vi "FlexDDS-NG_USB_Example.vi"() -> ()   [LabVIEW 2016]
uses:
  <vilib>/Utility/xml.llb/Read From XML File(string).vi
  <vilib>/Utility/xml.llb/Write to XML File(string).vi
panel:
  in  "appended instruction string 5":string="dds reset\rdcp spi:CFR1=0x404000\rdcp spi:CFR2=0x80080\rdcp 0 spi:STP0=0x3FFF0000028F5C29\rdcp 1 spi:STP0=0x3FFF0000028F5C29\rdcp 0 spi:DRL=0x147C0118147BC1DB\rdcp 0 spi:DRSS=0xFFFFFFFF00000003\rdcp 0 spi:DRR=0x2D3E\rdcp 0 update:u-d\rdcp 0 update:+d\rdcp 1 spi:DRL=0x147AE148147AE148\rdcp 1 spi:DRSS=0xFFFFFFFF00000000\rdcp 1 spi:DRR=0xFFFF\rdcp 1 update:u-d\rdcp 1 update:+d\rdcp wait:1h:\rdcp wait::DROVER\rdcp 0 spi:DRL=0x147C51F1147C0118\rdcp 0 spi:DRSS=0xFFFFFFFF00000004\rdcp 0 spi:DRR=0x2F2F\rdcp 0 update:u-d\rdcp 0 update:+d\rdcp wait:1h:\rdcp wait::DROVER\rdcp 0 spi:DRL=0x147CB92D147C51F1\rdcp 0 spi:DRSS=0xFFFFFFFF00000017\rdcp 0 spi:DRR=0xD478\rdcp 0 update:u-d\rdcp 0 update:+d\rdcp wait:1h:\rdcp wait::DROVER\rdcp 0 spi:DRL=0x147D3CCC147CB92D\rdcp 0 spi:DRSS=0xFFFFFFFF00000009\rdcp 0 spi:DRR=0x4136\rdcp 0 update:u-d\rdcp 0 update:+d\rdcp wait:1h:\rdcp wait::DROVER\rdcp 0 spi:DRL=0x147DE446147D3CCC\rdcp 0 spi:DRSS=0xFFFFFFFF0000000D\rdcp 0 spi:DRR=0x4A07\rdcp 0 update:u-d\rdcp 0 update:+d\rdcp wait:1h:\rdcp wait::DROVER\rdcp 0 spi:DRL=0x147EB8D6147DE446\rdcp 0 spi:DRSS=0xFFFFFFFF0000002B\rdcp 0 spi:DRR=0xC0EC\rdcp 0 update:u-d\rdcp 0 update:+d\rdcp wait:1h:\rdcp wait::DROVER\rdcp 0 spi:DRL=0x147FC5C3147EB8D6\rdcp 0 spi:DRSS=0xFFFFFFFF00000006\rdcp 0 spi:DRR=0x1547\rdcp 0 update:u-d\rdcp 0 update:+d\rdcp wait:1h:\rdcp wait::DROVER\rdcp 0 spi:DRL=0x148118A1147FC5C3\rdcp 0 spi:DRSS=0xFFFFFFFF0000001C\rdcp 0 spi:DRR=0x4ECD\rdcp 0 update:u-d\rdcp 0 update:+d\rdcp wait:1h:\rdcp wait::DROVER\rdcp 0 spi:DRL=0x1482C174148118A1\rdcp 0 spi:DRSS=0xFFFFFFFF00000049\rdcp 0 spi:DRR=0xA3E0\rdcp 0 update:u-d\rdcp 0 update:+d\rdcp wait:1h:\rdcp wait::DROVER\rdcp 0 spi:DRL=0x1484D2A81482C174\rdcp 0 spi:DRSS=0xFFFFFFFF00000003\rdcp 0 spi:DRR=0x568\rdcp 0 update:u-d\rdcp 0 update:+d\rdcp wait:1h:\rdcp wait::DROVER\rdcp 0 spi:DRL=0x148760AD1484D2A8\rdcp 0 spi:DRSS=0xFFFFFFFF0000008C\rdcp 0 spi:DRR=0xCC25\rdcp 0 update:u-d\rdcp 0 update:+d\rdcp wait:1h:\rdcp wait::DROVER\rdcp 0 spi:DRL=0x148A8111148760AD\rdcp 0 spi:DRSS=0xFFFFFFFF00000049\rdcp 0 spi:DRR=0x56FB\rdcp 0 update:u-d\rdcp 0 update:+d\rdcp wait:1h:\rdcp wait::DROVER\rdcp 0 spi:DRL=0x148E48EB148A8111\rdcp 0 spi:DRSS=0xFFFFFFFF00000004\rdcp 0 spi:DRR=0x3F1\rdcp 0 update:u-d\rdcp 0 update:+d\rdcp wait:1h:\rdcp wait::DROVER\rdcp 0 spi:DRL=0x1492CA77148E48EB\rdcp 0 spi:DRSS=0xFFFFFFFF000000A0\rdcp 0 spi:DRR=0x8447\rdcp 0 update:u-d\rdcp 0 update:+d\rdcp wait:1h:\rdcp wait::DROVER\rdcp 0 spi:DRL=0x149811DB1492CA77\rdcp 0 spi:DRSS=0xFFFFFFFF000000D0\rdcp 0 spi:DRR=0x92C9\rdcp 0 update:u-d\rdcp 0 update:+d\rdcp wait:1h:\rdcp wait::DROVER\rdcp 0 spi:DRL=0x149E2175149811DB\rdcp 0 spi:DRSS=0xFFFFFFFF00000100\rdcp 0 spi:DRR=0x9D59\rdcp 0 update:u-d\rdcp 0 update:+d\rdcp wait:1h:\rdcp wait::DROVER\rdcp 0 spi:DRL=0x14A4EE42149E2175\rdcp 0 spi:DRSS=0xFFFFFFFF000000C7\rdcp 0 spi:DRR=0x6D05\rdcp 0 update:u-d\rdcp 0 update:+d\rdcp wait:1h:\rdcp wait::DROVER\rdcp 0 spi:DRL=0x14AC5D7114A4EE42\rdcp 0 spi:DRSS=0xFFFFFFFF00000019\rdcp 0 spi:DRR=0xC87\rdcp 0 update:u-d\rdcp 0 update:+d\rdcp wait:1h:\rdcp wait::DROVER\rdcp 0 spi:DRL=0x14B4443314AC5D71\rdcp 0 spi:DRSS=0xFFFFFFFF00000021\rdcp 0 spi:DRR=0xF8F\rdcp 0 update:u-d\rdcp 0 update:+d\rdcp wait:1h:\rdcp wait::DROVER\rdcp 0 spi:DRL=0x14BC6A7F14B44433\rdcp 0 spi:DRSS=0xFFFFFFFF0000014D\rdcp 0 spi:DRR=0x9838\rdcp 0 update:u-d\rdcp 0 update:+d\rdcp wait:1h:\rdcp wait::DROVER\rdcp 0 spi:DRL=0x14C490CB14BC6A7F\rdcp 0 spi:DRSS=0xFFFFFFFF0000014D\rdcp 0 spi:DRR=0x9838\rdcp 0 update:u-d\rdcp 0 update:+d\rdcp wait:1h:\rdcp wait::DROVER\rdcp 0 spi:DRL=0x14CC778D14C490CB\rdcp 0 spi:DRSS=0xFFFFFFFF00000021\rdcp 0 spi:DRR=0xF8F\rdcp 0 update:u-d\rdcp 0 update:+d\rdcp wait:1h:\rdcp wait::DROVER\rdcp 0 spi:DRL=0x14D3E6BC14CC778D\rdcp 0 spi:DRSS=0xFFFFFFFF00000019\rdcp 0 spi:DRR=0xC87\rdcp 0 update:u-d\rdcp 0 update:+d\rdcp wait:1h:\rdcp wait::DROVER\rdcp 0 spi:DRL=0x14DAB38914D3E6BC\rdcp 0 spi:DRSS=0xFFFFFFFF000000C7\rdcp 0 spi:DRR=0x6D05\rdcp 0 update:u-d\rdcp 0 update:+d\rdcp wait:1h:\rdcp wait::DROVER\rdcp 0 spi:DRL=0x14E0C32314DAB389\rdcp 0 spi:DRSS=0xFFFFFFFF00000100\rdcp 0 spi:DRR=0x9D59\rdcp 0 update:u-d\rdcp 0 update:+d\rdcp wait:1h:\rdcp wait::DROVER\rdcp 0 spi:DRL=0x14E60A8714E0C323\rdcp 0 spi:DRSS=0xFFFFFFFF000000D0\rdcp 0 spi:DRR=0x92C9\rdcp 0 update:u-d\rdcp 0 update:+d\rdcp wait:1h:\rdcp wait::DROVER\rdcp 0 spi:DRL=0x14EA8C1314E60A87\rdcp 0 spi:DRSS=0xFFFFFFFF000000A0\rdcp 0 spi:DRR=0x8447\rdcp 0 update:u-d\rdcp 0 update:+d\rdcp wait:1h:\rdcp wait::DROVER\rdcp 0 spi:DRL=0x14EE53ED14EA8C13\rdcp 0 spi:DRSS=0xFFFFFFFF00000004\rdcp 0 spi:DRR=0x3F1\rdcp 0 update:u-d\rdcp 0 update:+d\rdcp wait:1h:\rdcp wait::DROVER\rdcp 0 spi:DRL=0x14F1745114EE53ED\rdcp 0 spi:DRSS=0xFFFFFFFF00000049\rdcp 0 spi:DRR=0x56FB\rdcp 0 update:u-d\rdcp 0 update:+d\rdcp wait:1h:\rdcp wait::DROVER\rdcp 0 spi:DRL=0x14F4025514F17451\rdcp 0 spi:DRSS=0xFFFFFFFF0000008C\rdcp 0 spi:DRR=0xCC25\rdcp 0 update:u-d\rdcp 0 update:+d\rdcp wait:1h:\rdcp wait::DROVER\rdcp 0 spi:DRL=0x14F6138A14F40255\rdcp 0 spi:DRSS=0xFFFFFFFF00000003\rdcp 0 spi:DRR=0x568\rdcp 0 update:u-d\rdcp 0 update:+d\rdcp wait:1h:\rdcp wait::DROVER\rdcp 0 spi:DRL=0x14F7BC5D14F6138A\rdcp 0 spi:DRSS=0xFFFFFFFF00000049\rdcp 0 spi:DRR=0xA3E0\rdcp 0 update:u-d\rdcp 0 update:+d\rdcp wait:1h:\rdcp wait::DROVER\rdcp 0 spi:DRL=0x14F90F3B14F7BC5D\rdcp 0 spi:DRSS=0xFFFFFFFF0000001C\rdcp 0 spi:DRR=0x4ECD\rdcp 0 update:u-d\rdcp 0 update:+d\rdcp wait:1h:\rdcp wait::DROVER\rdcp 0 spi:DRL=0x14FA1C2814F90F3B\rdcp 0 spi:DRSS=0xFFFFFFFF00000006\rdcp 0 spi:DRR=0x1547\rdcp 0 update:u-d\rdcp 0 update:+d\rdcp wait:1h:\rdcp wait::DROVER\rdcp 0 spi:DRL=0x14FAF0B814FA1C28\rdcp 0 spi:DRSS=0xFFFFFFFF0000002B\rdcp 0 spi:DRR=0xC0EC\rdcp 0 update:u-d\rdcp 0 update:+d\rdcp wait:1h:\rdcp wait::DROVER\rdcp 0 spi:DRL=0x14FB983214FAF0B8\rdcp 0 spi:DRSS=0xFFFFFFFF0000000D\rdcp 0 spi:DRR=0x4A07\rdcp 0 update:u-d\rdcp 0 update:+d\rdcp wait:1h:\rdcp wait::DROVER\rdcp 0 spi:DRL=0x14FC1BD114FB9832\rdcp 0 spi:DRSS=0xFFFFFFFF00000009\rdcp 0 spi:DRR=0x4136\rdcp 0 update:u-d\rdcp 0 update:+d\rdcp wait:1h:\rdcp wait::DROVER\rdcp 0 spi:DRL=0x14FC830D14FC1BD1\rdcp 0 spi:DRSS=0xFFFFFFFF00000017\rdcp 0 spi:DRR=0xD478\rdcp 0 update:u-d\rdcp 0 update:+d\rdcp wait:1h:\rdcp wait::DROVER\rdcp 0 spi:DRL=0x14FCD3E614FC830D\rdcp 0 spi:DRSS=0xFFFFFFFF00000004\rdcp 0 spi:DRR=0x2F2F\rdcp 0 update:u-d\rdcp 0 update:+d\rdcp wait:1h:\rdcp wait::DROVER\rdcp 0 spi:DRL=0x14FD132314FCD3E6\rdcp 0 spi:DRSS=0xFFFFFFFF00000003\rdcp 0 spi:DRR=0x2D3E\rdcp 0 update:u-d\rdcp 0 update:+d\rdcp wait:1h:\rdcp wait::DROVER\rdcp 0 spi:DRL=0x14FD448E14FD1323\rdcp 0 spi:DRSS=0xFFFFFFFF00000002\rdcp 0 spi:DRR=0x2699\rdcp 0 update:u-d\rdcp 0 update:+d\rdcp wait:1h:\rdcp wait::DROVER\rdcp start\r"
  out "appended instruction string 4":string="dds reset\rdcp spi:CFR1=0x404000\rdcp spi:CFR2=0x80080\rdcp 0 spi:STP0=0x3FFF0000028F5C29\rdcp 1 spi:STP0=0x3FFF0000028F5C29\rdcp 0 spi:DRL=0x147C0118147BC1DB\rdcp 0 spi:DRSS=0xFFFFFFFF00000003\rdcp 0 spi:DRR=0x2D3E\rdcp 0 update:u-d\rdcp 0 update:+d\rdcp 1 spi:DRL=0x147AE148147AE148\rdcp 1 spi:DRSS=0xFFFFFFFF00000000\rdcp 1 spi:DRR=0xFFFF\rdcp 1 update:u-d\rdcp 1 update:+d\rdcp wait:1h:\rdcp wait::DROVER\rdcp 0 spi:DRL=0x147C51F1147C0118\rdcp 0 spi:DRSS=0xFFFFFFFF00000004\rdcp 0 spi:DRR=0x2F2F\rdcp 0 update:u-d\rdcp 0 update:+d\rdcp wait:1h:\rdcp wait::DROVER\rdcp 0 spi:DRL=0x147CB92D147C51F1\rdcp 0 spi:DRSS=0xFFFFFFFF00000017\rdcp 0 spi:DRR=0xD478\rdcp 0 update:u-d\rdcp 0 update:+d\rdcp wait:1h:\rdcp wait::DROVER\rdcp 0 spi:DRL=0x147D3CCC147CB92D\rdcp 0 spi:DRSS=0xFFFFFFFF00000009\rdcp 0 spi:DRR=0x4136\rdcp 0 update:u-d\rdcp 0 update:+d\rdcp wait:1h:\rdcp wait::DROVER\rdcp 0 spi:DRL=0x147DE446147D3CCC\rdcp 0 spi:DRSS=0xFFFFFFFF0000000D\rdcp 0 spi:DRR=0x4A07\rdcp 0 update:u-d\rdcp 0 update:+d\rdcp wait:1h:\rdcp wait::DROVER\rdcp 0 spi:DRL=0x147EB8D6147DE446\rdcp 0 spi:DRSS=0xFFFFFFFF0000002B\rdcp 0 spi:DRR=0xC0EC\rdcp 0 update:u-d\rdcp 0 update:+d\rdcp wait:1h:\rdcp wait::DROVER\rdcp 0 spi:DRL=0x147FC5C3147EB8D6\rdcp 0 spi:DRSS=0xFFFFFFFF00000006\rdcp 0 spi:DRR=0x1547\rdcp 0 update:u-d\rdcp 0 update:+d\rdcp wait:1h:\rdcp wait::DROVER\rdcp 0 spi:DRL=0x148118A1147FC5C3\rdcp 0 spi:DRSS=0xFFFFFFFF0000001C\rdcp 0 spi:DRR=0x4ECD\rdcp 0 update:u-d\rdcp 0 update:+d\rdcp wait:1h:\rdcp wait::DROVER\rdcp 0 spi:DRL=0x1482C174148118A1\rdcp 0 spi:DRSS=0xFFFFFFFF00000049\rdcp 0 spi:DRR=0xA3E0\rdcp 0 update:u-d\rdcp 0 update:+d\rdcp wait:1h:\rdcp wait::DROVER\rdcp 0 spi:DRL=0x1484D2A81482C174\rdcp 0 spi:DRSS=0xFFFFFFFF00000003\rdcp 0 spi:DRR=0x568\rdcp 0 update:u-d\rdcp 0 update:+d\rdcp wait:1h:\rdcp wait::DROVER\rdcp 0 spi:DRL=0x148760AD1484D2A8\rdcp 0 spi:DRSS=0xFFFFFFFF0000008C\rdcp 0 spi:DRR=0xCC25\rdcp 0 update:u-d\rdcp 0 update:+d\rdcp wait:1h:\rdcp wait::DROVER\rdcp 0 spi:DRL=0x148A8111148760AD\rdcp 0 spi:DRSS=0xFFFFFFFF00000049\rdcp 0 spi:DRR=0x56FB\rdcp 0 update:u-d\rdcp 0 update:+d\rdcp wait:1h:\rdcp wait::DROVER\rdcp 0 spi:DRL=0x148E48EB148A8111\rdcp 0 spi:DRSS=0xFFFFFFFF00000004\rdcp 0 spi:DRR=0x3F1\rdcp 0 update:u-d\rdcp 0 update:+d\rdcp wait:1h:\rdcp wait::DROVER\rdcp 0 spi:DRL=0x1492CA77148E48EB\rdcp 0 spi:DRSS=0xFFFFFFFF000000A0\rdcp 0 spi:DRR=0x8447\rdcp 0 update:u-d\rdcp 0 update:+d\rdcp wait:1h:\rdcp wait::DROVER\rdcp 0 spi:DRL=0x149811DB1492CA77\rdcp 0 spi:DRSS=0xFFFFFFFF000000D0\rdcp 0 spi:DRR=0x92C9\rdcp 0 update:u-d\rdcp 0 update:+d\rdcp wait:1h:\rdcp wait::DROVER\rdcp 0 spi:DRL=0x149E2175149811DB\rdcp 0 spi:DRSS=0xFFFFFFFF00000100\rdcp 0 spi:DRR=0x9D59\rdcp 0 update:u-d\rdcp 0 update:+d\rdcp wait:1h:\rdcp wait::DROVER\rdcp 0 spi:DRL=0x14A4EE42149E2175\rdcp 0 spi:DRSS=0xFFFFFFFF000000C7\rdcp 0 spi:DRR=0x6D05\rdcp 0 update:u-d\rdcp 0 update:+d\rdcp wait:1h:\rdcp wait::DROVER\rdcp 0 spi:DRL=0x14AC5D7114A4EE42\rdcp 0 spi:DRSS=0xFFFFFFFF00000019\rdcp 0 spi:DRR=0xC87\rdcp 0 update:u-d\rdcp 0 update:+d\rdcp wait:1h:\rdcp wait::DROVER\rdcp 0 spi:DRL=0x14B4443314AC5D71\rdcp 0 spi:DRSS=0xFFFFFFFF00000021\rdcp 0 spi:DRR=0xF8F\rdcp 0 update:u-d\rdcp 0 update:+d\rdcp wait:1h:\rdcp wait::DROVER\rdcp 0 spi:DRL=0x14BC6A7F14B44433\rdcp 0 spi:DRSS=0xFFFFFFFF0000014D\rdcp 0 spi:DRR=0x9838\rdcp 0 update:u-d\rdcp 0 update:+d\rdcp wait:1h:\rdcp wait::DROVER\rdcp 0 spi:DRL=0x14C490CB14BC6A7F\rdcp 0 spi:DRSS=0xFFFFFFFF0000014D\rdcp 0 spi:DRR=0x9838\rdcp 0 update:u-d\rdcp 0 update:+d\rdcp wait:1h:\rdcp wait::DROVER\rdcp 0 spi:DRL=0x14CC778D14C490CB\rdcp 0 spi:DRSS=0xFFFFFFFF00000021\rdcp 0 spi:DRR=0xF8F\rdcp 0 update:u-d\rdcp 0 update:+d\rdcp wait:1h:\rdcp wait::DROVER\rdcp 0 spi:DRL=0x14D3E6BC14CC778D\rdcp 0 spi:DRSS=0xFFFFFFFF00000019\rdcp 0 spi:DRR=0xC87\rdcp 0 update:u-d\rdcp 0 update:+d\rdcp wait:1h:\rdcp wait::DROVER\rdcp 0 spi:DRL=0x14DAB38914D3E6BC\rdcp 0 spi:DRSS=0xFFFFFFFF000000C7\rdcp 0 spi:DRR=0x6D05\rdcp 0 update:u-d\rdcp 0 update:+d\rdcp wait:1h:\rdcp wait::DROVER\rdcp 0 spi:DRL=0x14E0C32314DAB389\rdcp 0 spi:DRSS=0xFFFFFFFF00000100\rdcp 0 spi:DRR=0x9D59\rdcp 0 update:u-d\rdcp 0 update:+d\rdcp wait:1h:\rdcp wait::DROVER\rdcp 0 spi:DRL=0x14E60A8714E0C323\rdcp 0 spi:DRSS=0xFFFFFFFF000000D0\rdcp 0 spi:DRR=0x92C9\rdcp 0 update:u-d\rdcp 0 update:+d\rdcp wait:1h:\rdcp wait::DROVER\rdcp 0 spi:DRL=0x14EA8C1314E60A87\rdcp 0 spi:DRSS=0xFFFFFFFF000000A0\rdcp 0 spi:DRR=0x8447\rdcp 0 update:u-d\rdcp 0 update:+d\rdcp wait:1h:\rdcp wait::DROVER\rdcp 0 spi:DRL=0x14EE53ED14EA8C13\rdcp 0 spi:DRSS=0xFFFFFFFF00000004\rdcp 0 spi:DRR=0x3F1\rdcp 0 update:u-d\rdcp 0 update:+d\rdcp wait:1h:\rdcp wait::DROVER\rdcp 0 spi:DRL=0x14F1745114EE53ED\rdcp 0 spi:DRSS=0xFFFFFFFF00000049\rdcp 0 spi:DRR=0x56FB\rdcp 0 update:u-d\rdcp 0 update:+d\rdcp wait:1h:\rdcp wait::DROVER\rdcp 0 spi:DRL=0x14F4025514F17451\rdcp 0 spi:DRSS=0xFFFFFFFF0000008C\rdcp 0 spi:DRR=0xCC25\rdcp 0 update:u-d\rdcp 0 update:+d\rdcp wait:1h:\rdcp wait::DROVER\rdcp 0 spi:DRL=0x14F6138A14F40255\rdcp 0 spi:DRSS=0xFFFFFFFF00000003\rdcp 0 spi:DRR=0x568\rdcp 0 update:u-d\rdcp 0 update:+d\rdcp wait:1h:\rdcp wait::DROVER\rdcp 0 spi:DRL=0x14F7BC5D14F6138A\rdcp 0 spi:DRSS=0xFFFFFFFF00000049\rdcp 0 spi:DRR=0xA3E0\rdcp 0 update:u-d\rdcp 0 update:+d\rdcp wait:1h:\rdcp wait::DROVER\rdcp 0 spi:DRL=0x14F90F3B14F7BC5D\rdcp 0 spi:DRSS=0xFFFFFFFF0000001C\rdcp 0 spi:DRR=0x4ECD\rdcp 0 update:u-d\rdcp 0 update:+d\rdcp wait:1h:\rdcp wait::DROVER\rdcp 0 spi:DRL=0x14FA1C2814F90F3B\rdcp 0 spi:DRSS=0xFFFFFFFF00000006\rdcp 0 spi:DRR=0x1547\rdcp 0 update:u-d\rdcp 0 update:+d\rdcp wait:1h:\rdcp wait::DROVER\rdcp 0 spi:DRL=0x14FAF0B814FA1C28\rdcp 0 spi:DRSS=0xFFFFFFFF0000002B\rdcp 0 spi:DRR=0xC0EC\rdcp 0 update:u-d\rdcp 0 update:+d\rdcp wait:1h:\rdcp wait::DROVER\rdcp 0 spi:DRL=0x14FB983214FAF0B8\rdcp 0 spi:DRSS=0xFFFFFFFF0000000D\rdcp 0 spi:DRR=0x4A07\rdcp 0 update:u-d\rdcp 0 update:+d\rdcp wait:1h:\rdcp wait::DROVER\rdcp 0 spi:DRL=0x14FC1BD114FB9832\rdcp 0 spi:DRSS=0xFFFFFFFF00000009\rdcp 0 spi:DRR=0x4136\rdcp 0 update:u-d\rdcp 0 update:+d\rdcp wait:1h:\rdcp wait::DROVER\rdcp 0 spi:DRL=0x14FC830D14FC1BD1\rdcp 0 spi:DRSS=0xFFFFFFFF00000017\rdcp 0 spi:DRR=0xD478\rdcp 0 update:u-d\rdcp 0 update:+d\rdcp wait:1h:\rdcp wait::DROVER\rdcp 0 spi:DRL=0x14FCD3E614FC830D\rdcp 0 spi:DRSS=0xFFFFFFFF00000004\rdcp 0 spi:DRR=0x2F2F\rdcp 0 update:u-d\rdcp 0 update:+d\rdcp wait:1h:\rdcp wait::DROVER\rdcp 0 spi:DRL=0x14FD132314FCD3E6\rdcp 0 spi:DRSS=0xFFFFFFFF00000003\rdcp 0 spi:DRR=0x2D3E\rdcp 0 update:u-d\rdcp 0 update:+d\rdcp wait:1h:\rdcp wait::DROVER\rdcp 0 spi:DRL=0x14FD448E14FD1323\rdcp 0 spi:DRSS=0xFFFFFFFF00000002\rdcp 0 spi:DRR=0x2699\rdcp 0 update:u-d\rdcp 0 update:+d\rdcp wait:1h:\rdcp wait::DROVER\rdcp start\r"
  in  "appended instruction string 3":string="dds reset\rdcp spi:CFR1=0x404000\rdcp spi:CFR2=0x80080\rdcp 0 spi:STP0=0x3FFF0000028F5C29\rdcp 1 spi:STP0=0x3FFF0000028F5C29\rdcp 0 spi:DRL=0x147C0118147BC1DB\rdcp 0 spi:DRSS=0xFFFFFFFF00000003\rdcp 0 spi:DRR=0x2D3E\rdcp 0 update:u-d\rdcp 0 update:+d\rdcp 1 spi:DRL=0x147AE148147AE148\rdcp 1 spi:DRSS=0xFFFFFFFF00000000\rdcp 1 spi:DRR=0xFFFF\rdcp 1 update:u-d\rdcp 1 update:+d\rdcp wait:1h:\rdcp wait::DROVER\rdcp 0 spi:DRL=0x147C51F1147C0118\rdcp 0 spi:DRSS=0xFFFFFFFF00000004\rdcp 0 spi:DRR=0x2F2F\rdcp 0 update:u-d\rdcp 0 update:+d\rdcp wait:1h:\rdcp wait::DROVER\rdcp 0 spi:DRL=0x147CB92D147C51F1\rdcp 0 spi:DRSS=0xFFFFFFFF00000017\rdcp 0 spi:DRR=0xD478\rdcp 0 update:u-d\rdcp 0 update:+d\rdcp wait:1h:\rdcp wait::DROVER\rdcp 0 spi:DRL=0x147D3CCC147CB92D\rdcp 0 spi:DRSS=0xFFFFFFFF00000009\rdcp 0 spi:DRR=0x4136\rdcp 0 update:u-d\rdcp 0 update:+d\rdcp wait:1h:\rdcp wait::DROVER\rdcp 0 spi:DRL=0x147DE446147D3CCC\rdcp 0 spi:DRSS=0xFFFFFFFF0000000D\rdcp 0 spi:DRR=0x4A07\rdcp 0 update:u-d\rdcp 0 update:+d\rdcp wait:1h:\rdcp wait::DROVER\rdcp 0 spi:DRL=0x147EB8D6147DE446\rdcp 0 spi:DRSS=0xFFFFFFFF0000002B\rdcp 0 spi:DRR=0xC0EC\rdcp 0 update:u-d\rdcp 0 update:+d\rdcp wait:1h:\rdcp wait::DROVER\rdcp 0 spi:DRL=0x147FC5C3147EB8D6\rdcp 0 spi:DRSS=0xFFFFFFFF00000006\rdcp 0 spi:DRR=0x1547\rdcp 0 update:u-d\rdcp 0 update:+d\rdcp wait:1h:\rdcp wait::DROVER\rdcp 0 spi:DRL=0x148118A1147FC5C3\rdcp 0 spi:DRSS=0xFFFFFFFF0000001C\rdcp 0 spi:DRR=0x4ECD\rdcp 0 update:u-d\rdcp 0 update:+d\rdcp wait:1h:\rdcp wait::DROVER\rdcp 0 spi:DRL=0x1482C174148118A1\rdcp 0 spi:DRSS=0xFFFFFFFF00000049\rdcp 0 spi:DRR=0xA3E0\rdcp 0 update:u-d\rdcp 0 update:+d\rdcp wait:1h:\rdcp wait::DROVER\rdcp 0 spi:DRL=0x1484D2A81482C174\rdcp 0 spi:DRSS=0xFFFFFFFF00000003\rdcp 0 spi:DRR=0x568\rdcp 0 update:u-d\rdcp 0 update:+d\rdcp wait:1h:\rdcp wait::DROVER\rdcp 0 spi:DRL=0x148760AD1484D2A8\rdcp 0 spi:DRSS=0xFFFFFFFF0000008C\rdcp 0 spi:DRR=0xCC25\rdcp 0 update:u-d\rdcp 0 update:+d\rdcp wait:1h:\rdcp wait::DROVER\rdcp 0 spi:DRL=0x148A8111148760AD\rdcp 0 spi:DRSS=0xFFFFFFFF00000049\rdcp 0 spi:DRR=0x56FB\rdcp 0 update:u-d\rdcp 0 update:+d\rdcp wait:1h:\rdcp wait::DROVER\rdcp 0 spi:DRL=0x148E48EB148A8111\rdcp 0 spi:DRSS=0xFFFFFFFF00000004\rdcp 0 spi:DRR=0x3F1\rdcp 0 update:u-d\rdcp 0 update:+d\rdcp wait:1h:\rdcp wait::DROVER\rdcp 0 spi:DRL=0x1492CA77148E48EB\rdcp 0 spi:DRSS=0xFFFFFFFF000000A0\rdcp 0 spi:DRR=0x8447\rdcp 0 update:u-d\rdcp 0 update:+d\rdcp wait:1h:\rdcp wait::DROVER\rdcp 0 spi:DRL=0x149811DB1492CA77\rdcp 0 spi:DRSS=0xFFFFFFFF000000D0\rdcp 0 spi:DRR=0x92C9\rdcp 0 update:u-d\rdcp 0 update:+d\rdcp wait:1h:\rdcp wait::DROVER\rdcp 0 spi:DRL=0x149E2175149811DB\rdcp 0 spi:DRSS=0xFFFFFFFF00000100\rdcp 0 spi:DRR=0x9D59\rdcp 0 update:u-d\rdcp 0 update:+d\rdcp wait:1h:\rdcp wait::DROVER\rdcp 0 spi:DRL=0x14A4EE42149E2175\rdcp 0 spi:DRSS=0xFFFFFFFF000000C7\rdcp 0 spi:DRR=0x6D05\rdcp 0 update:u-d\rdcp 0 update:+d\rdcp wait:1h:\rdcp wait::DROVER\rdcp 0 spi:DRL=0x14AC5D7114A4EE42\rdcp 0 spi:DRSS=0xFFFFFFFF00000019\rdcp 0 spi:DRR=0xC87\rdcp 0 update:u-d\rdcp 0 update:+d\rdcp wait:1h:\rdcp wait::DROVER\rdcp 0 spi:DRL=0x14B4443314AC5D71\rdcp 0 spi:DRSS=0xFFFFFFFF00000021\rdcp 0 spi:DRR=0xF8F\rdcp 0 update:u-d\rdcp 0 update:+d\rdcp wait:1h:\rdcp wait::DROVER\rdcp 0 spi:DRL=0x14BC6A7F14B44433\rdcp 0 spi:DRSS=0xFFFFFFFF0000014D\rdcp 0 spi:DRR=0x9838\rdcp 0 update:u-d\rdcp 0 update:+d\rdcp wait:1h:\rdcp wait::DROVER\rdcp 0 spi:DRL=0x14C490CB14BC6A7F\rdcp 0 spi:DRSS=0xFFFFFFFF0000014D\rdcp 0 spi:DRR=0x9838\rdcp 0 update:u-d\rdcp 0 update:+d\rdcp wait:1h:\rdcp wait::DROVER\rdcp 0 spi:DRL=0x14CC778D14C490CB\rdcp 0 spi:DRSS=0xFFFFFFFF00000021\rdcp 0 spi:DRR=0xF8F\rdcp 0 update:u-d\rdcp 0 update:+d\rdcp wait:1h:\rdcp wait::DROVER\rdcp 0 spi:DRL=0x14D3E6BC14CC778D\rdcp 0 spi:DRSS=0xFFFFFFFF00000019\rdcp 0 spi:DRR=0xC87\rdcp 0 update:u-d\rdcp 0 update:+d\rdcp wait:1h:\rdcp wait::DROVER\rdcp 0 spi:DRL=0x14DAB38914D3E6BC\rdcp 0 spi:DRSS=0xFFFFFFFF000000C7\rdcp 0 spi:DRR=0x6D05\rdcp 0 update:u-d\rdcp 0 update:+d\rdcp wait:1h:\rdcp wait::DROVER\rdcp 0 spi:DRL=0x14E0C32314DAB389\rdcp 0 spi:DRSS=0xFFFFFFFF00000100\rdcp 0 spi:DRR=0x9D59\rdcp 0 update:u-d\rdcp 0 update:+d\rdcp wait:1h:\rdcp wait::DROVER\rdcp 0 spi:DRL=0x14E60A8714E0C323\rdcp 0 spi:DRSS=0xFFFFFFFF000000D0\rdcp 0 spi:DRR=0x92C9\rdcp 0 update:u-d\rdcp 0 update:+d\rdcp wait:1h:\rdcp wait::DROVER\rdcp 0 spi:DRL=0x14EA8C1314E60A87\rdcp 0 spi:DRSS=0xFFFFFFFF000000A0\rdcp 0 spi:DRR=0x8447\rdcp 0 update:u-d\rdcp 0 update:+d\rdcp wait:1h:\rdcp wait::DROVER\rdcp 0 spi:DRL=0x14EE53ED14EA8C13\rdcp 0 spi:DRSS=0xFFFFFFFF00000004\rdcp 0 spi:DRR=0x3F1\rdcp 0 update:u-d\rdcp 0 update:+d\rdcp wait:1h:\rdcp wait::DROVER\rdcp 0 spi:DRL=0x14F1745114EE53ED\rdcp 0 spi:DRSS=0xFFFFFFFF00000049\rdcp 0 spi:DRR=0x56FB\rdcp 0 update:u-d\rdcp 0 update:+d\rdcp wait:1h:\rdcp wait::DROVER\rdcp 0 spi:DRL=0x14F4025514F17451\rdcp 0 spi:DRSS=0xFFFFFFFF0000008C\rdcp 0 spi:DRR=0xCC25\rdcp 0 update:u-d\rdcp 0 update:+d\rdcp wait:1h:\rdcp wait::DROVER\rdcp 0 spi:DRL=0x14F6138A14F40255\rdcp 0 spi:DRSS=0xFFFFFFFF00000003\rdcp 0 spi:DRR=0x568\rdcp 0 update:u-d\rdcp 0 update:+d\rdcp wait:1h:\rdcp wait::DROVER\rdcp 0 spi:DRL=0x14F7BC5D14F6138A\rdcp 0 spi:DRSS=0xFFFFFFFF00000049\rdcp 0 spi:DRR=0xA3E0\rdcp 0 update:u-d\rdcp 0 update:+d\rdcp wait:1h:\rdcp wait::DROVER\rdcp 0 spi:DRL=0x14F90F3B14F7BC5D\rdcp 0 spi:DRSS=0xFFFFFFFF0000001C\rdcp 0 spi:DRR=0x4ECD\rdcp 0 update:u-d\rdcp 0 update:+d\rdcp wait:1h:\rdcp wait::DROVER\rdcp 0 spi:DRL=0x14FA1C2814F90F3B\rdcp 0 spi:DRSS=0xFFFFFFFF00000006\rdcp 0 spi:DRR=0x1547\rdcp 0 update:u-d\rdcp 0 update:+d\rdcp wait:1h:\rdcp wait::DROVER\rdcp 0 spi:DRL=0x14FAF0B814FA1C28\rdcp 0 spi:DRSS=0xFFFFFFFF0000002B\rdcp 0 spi:DRR=0xC0EC\rdcp 0 update:u-d\rdcp 0 update:+d\rdcp wait:1h:\rdcp wait::DROVER\rdcp 0 spi:DRL=0x14FB983214FAF0B8\rdcp 0 spi:DRSS=0xFFFFFFFF0000000D\rdcp 0 spi:DRR=0x4A07\rdcp 0 update:u-d\rdcp 0 update:+d\rdcp wait:1h:\rdcp wait::DROVER\rdcp 0 spi:DRL=0x14FC1BD114FB9832\rdcp 0 spi:DRSS=0xFFFFFFFF00000009\rdcp 0 spi:DRR=0x4136\rdcp 0 update:u-d\rdcp 0 update:+d\rdcp wait:1h:\rdcp wait::DROVER\rdcp 0 spi:DRL=0x14FC830D14FC1BD1\rdcp 0 spi:DRSS=0xFFFFFFFF00000017\rdcp 0 spi:DRR=0xD478\rdcp 0 update:u-d\rdcp 0 update:+d\rdcp wait:1h:\rdcp wait::DROVER\rdcp 0 spi:DRL=0x14FCD3E614FC830D\rdcp 0 spi:DRSS=0xFFFFFFFF00000004\rdcp 0 spi:DRR=0x2F2F\rdcp 0 update:u-d\rdcp 0 update:+d\rdcp wait:1h:\rdcp wait::DROVER\rdcp 0 spi:DRL=0x14FD132314FCD3E6\rdcp 0 spi:DRSS=0xFFFFFFFF00000003\rdcp 0 spi:DRR=0x2D3E\rdcp 0 update:u-d\rdcp 0 update:+d\rdcp wait:1h:\rdcp wait::DROVER\rdcp 0 spi:DRL=0x14FD448E14FD1323\rdcp 0 spi:DRSS=0xFFFFFFFF00000002\rdcp 0 spi:DRR=0x2699\rdcp 0 update:u-d\rdcp 0 update:+d\rdcp wait:1h:\rdcp wait::DROVER\rdcp start\r"
  in  "Interactive on/off":T1(ring)
  out "return count":u32=6435
  in  "Store data":enum32{"Save settings", "Don't save settings"}(tab)=enum."Don't save settings"
  in  "XML File Path WRITE":path=path "U:/Dokumente/Bachelorarbeit/Labview/FlexDDS-NG/conf/settings_s_curve_up_down.xml"
  in  "Data source":T2(tab)=enum."Generate data with function"
  in  "XML File Path READ":path=path "U:/Dokumente/Bachelorarbeit/Labview/FlexDDS-NG/conf/settings_4consecutive_falling.xml"
  in  "Select curve form":enum32{"S curve", "Exp curve"}(tab)
  in  "s curve parameters":cluster{"k":dbl}={"k"=10.0}
  in  "exp curve parameters":cluster{"k":dbl}={"k"=5.0}
  in  "parameters non-constant channel":T3={"Number of steps"=40, "time [ms]"=10000.0, "start frequency [Hz]"=80000000.0, "end frequency [Hz]"=82000000.0}
  in  "constant frequency":dbl=80000000.0 format="%#_13g"
  in  "Constant Channel":T4(ring)
  in  "CFR2 bits":T5={"Enable ASF from STP (F)"=FALSE, "Digital ramp enable (F)"=TRUE, "Digital ramp no-dwell high (F)"=FALSE, "Digital ramp no-dwell low (F)"=FALSE, "Matched latency enable (T)"=TRUE, "Parallel data port enable (F)"=FALSE}
  in  "CFR1 bits":T6={"RAM enable (F)"=FALSE, "Manual OSK external control (F)"=FALSE, "Inverse sinc filter enable (T)"=TRUE, "DDS sine (/cosine) output (F)"=FALSE, "Load LRR at I/O update (F)"=FALSE, "Autoclear digital ramp accumulator (F)"=TRUE, "Autoclear phase accumulator (F)"=FALSE, "Clear digital ramp accumulator (F)"=FALSE, "Clear phase accumulator (F)"=FALSE, "Load ARR at I/O update (F)"=FALSE, "OSK enable (F)"=FALSE, "Select Auto OSK (F)"=FALSE}
  in  "Trigger before sequence of sweeps":T7(ring)
  in  "appended instruction string 2":string="dds reset\rdcp spi:CFR1=0x404000\rdcp spi:CFR2=0x80080\rdcp 0 spi:STP0=0x3FFF0000028F5C29\rdcp 1 spi:STP0=0x3FFF0000028F5C29\rdcp 0 spi:DRL=0x147C0118147BC1DB\rdcp 0 spi:DRSS=0xFFFFFFFF00000003\rdcp 0 spi:DRR=0x2D3E\rdcp 0 update:u-d\rdcp 0 update:+d\rdcp 1 spi:DRL=0x147AE148147AE148\rdcp 1 spi:DRSS=0xFFFFFFFF00000000\rdcp 1 spi:DRR=0xFFFF\rdcp 1 update:u-d\rdcp 1 update:+d\rdcp wait:1h:\rdcp wait::DROVER\rdcp 0 spi:DRL=0x147C51F1147C0118\rdcp 0 spi:DRSS=0xFFFFFFFF00000004\rdcp 0 spi:DRR=0x2F2F\rdcp 0 update:u-d\rdcp 0 update:+d\rdcp wait:1h:\rdcp wait::DROVER\rdcp 0 spi:DRL=0x147CB92D147C51F1\rdcp 0 spi:DRSS=0xFFFFFFFF00000017\rdcp 0 spi:DRR=0xD478\rdcp 0 update:u-d\rdcp 0 update:+d\rdcp wait:1h:\rdcp wait::DROVER\rdcp 0 spi:DRL=0x147D3CCC147CB92D\rdcp 0 spi:DRSS=0xFFFFFFFF00000009\rdcp 0 spi:DRR=0x4136\rdcp 0 update:u-d\rdcp 0 update:+d\rdcp wait:1h:\rdcp wait::DROVER\rdcp 0 spi:DRL=0x147DE446147D3CCC\rdcp 0 spi:DRSS=0xFFFFFFFF0000000D\rdcp 0 spi:DRR=0x4A07\rdcp 0 update:u-d\rdcp 0 update:+d\rdcp wait:1h:\rdcp wait::DROVER\rdcp 0 spi:DRL=0x147EB8D6147DE446\rdcp 0 spi:DRSS=0xFFFFFFFF0000002B\rdcp 0 spi:DRR=0xC0EC\rdcp 0 update:u-d\rdcp 0 update:+d\rdcp wait:1h:\rdcp wait::DROVER\rdcp 0 spi:DRL=0x147FC5C3147EB8D6\rdcp 0 spi:DRSS=0xFFFFFFFF00000006\rdcp 0 spi:DRR=0x1547\rdcp 0 update:u-d\rdcp 0 update:+d\rdcp wait:1h:\rdcp wait::DROVER\rdcp 0 spi:DRL=0x148118A1147FC5C3\rdcp 0 spi:DRSS=0xFFFFFFFF0000001C\rdcp 0 spi:DRR=0x4ECD\rdcp 0 update:u-d\rdcp 0 update:+d\rdcp wait:1h:\rdcp wait::DROVER\rdcp 0 spi:DRL=0x1482C174148118A1\rdcp 0 spi:DRSS=0xFFFFFFFF00000049\rdcp 0 spi:DRR=0xA3E0\rdcp 0 update:u-d\rdcp 0 update:+d\rdcp wait:1h:\rdcp wait::DROVER\rdcp 0 spi:DRL=0x1484D2A81482C174\rdcp 0 spi:DRSS=0xFFFFFFFF00000003\rdcp 0 spi:DRR=0x568\rdcp 0 update:u-d\rdcp 0 update:+d\rdcp wait:1h:\rdcp wait::DROVER\rdcp 0 spi:DRL=0x148760AD1484D2A8\rdcp 0 spi:DRSS=0xFFFFFFFF0000008C\rdcp 0 spi:DRR=0xCC25\rdcp 0 update:u-d\rdcp 0 update:+d\rdcp wait:1h:\rdcp wait::DROVER\rdcp 0 spi:DRL=0x148A8111148760AD\rdcp 0 spi:DRSS=0xFFFFFFFF00000049\rdcp 0 spi:DRR=0x56FB\rdcp 0 update:u-d\rdcp 0 update:+d\rdcp wait:1h:\rdcp wait::DROVER\rdcp 0 spi:DRL=0x148E48EB148A8111\rdcp 0 spi:DRSS=0xFFFFFFFF00000004\rdcp 0 spi:DRR=0x3F1\rdcp 0 update:u-d\rdcp 0 update:+d\rdcp wait:1h:\rdcp wait::DROVER\rdcp 0 spi:DRL=0x1492CA77148E48EB\rdcp 0 spi:DRSS=0xFFFFFFFF000000A0\rdcp 0 spi:DRR=0x8447\rdcp 0 update:u-d\rdcp 0 update:+d\rdcp wait:1h:\rdcp wait::DROVER\rdcp 0 spi:DRL=0x149811DB1492CA77\rdcp 0 spi:DRSS=0xFFFFFFFF000000D0\rdcp 0 spi:DRR=0x92C9\rdcp 0 update:u-d\rdcp 0 update:+d\rdcp wait:1h:\rdcp wait::DROVER\rdcp 0 spi:DRL=0x149E2175149811DB\rdcp 0 spi:DRSS=0xFFFFFFFF00000100\rdcp 0 spi:DRR=0x9D59\rdcp 0 update:u-d\rdcp 0 update:+d\rdcp wait:1h:\rdcp wait::DROVER\rdcp 0 spi:DRL=0x14A4EE42149E2175\rdcp 0 spi:DRSS=0xFFFFFFFF000000C7\rdcp 0 spi:DRR=0x6D05\rdcp 0 update:u-d\rdcp 0 update:+d\rdcp wait:1h:\rdcp wait::DROVER\rdcp 0 spi:DRL=0x14AC5D7114A4EE42\rdcp 0 spi:DRSS=0xFFFFFFFF00000019\rdcp 0 spi:DRR=0xC87\rdcp 0 update:u-d\rdcp 0 update:+d\rdcp wait:1h:\rdcp wait::DROVER\rdcp 0 spi:DRL=0x14B4443314AC5D71\rdcp 0 spi:DRSS=0xFFFFFFFF00000021\rdcp 0 spi:DRR=0xF8F\rdcp 0 update:u-d\rdcp 0 update:+d\rdcp wait:1h:\rdcp wait::DROVER\rdcp 0 spi:DRL=0x14BC6A7F14B44433\rdcp 0 spi:DRSS=0xFFFFFFFF0000014D\rdcp 0 spi:DRR=0x9838\rdcp 0 update:u-d\rdcp 0 update:+d\rdcp wait:1h:\rdcp wait::DROVER\rdcp 0 spi:DRL=0x14C490CB14BC6A7F\rdcp 0 spi:DRSS=0xFFFFFFFF0000014D\rdcp 0 spi:DRR=0x9838\rdcp 0 update:u-d\rdcp 0 update:+d\rdcp wait:1h:\rdcp wait::DROVER\rdcp 0 spi:DRL=0x14CC778D14C490CB\rdcp 0 spi:DRSS=0xFFFFFFFF00000021\rdcp 0 spi:DRR=0xF8F\rdcp 0 update:u-d\rdcp 0 update:+d\rdcp wait:1h:\rdcp wait::DROVER\rdcp 0 spi:DRL=0x14D3E6BC14CC778D\rdcp 0 spi:DRSS=0xFFFFFFFF00000019\rdcp 0 spi:DRR=0xC87\rdcp 0 update:u-d\rdcp 0 update:+d\rdcp wait:1h:\rdcp wait::DROVER\rdcp 0 spi:DRL=0x14DAB38914D3E6BC\rdcp 0 spi:DRSS=0xFFFFFFFF000000C7\rdcp 0 spi:DRR=0x6D05\rdcp 0 update:u-d\rdcp 0 update:+d\rdcp wait:1h:\rdcp wait::DROVER\rdcp 0 spi:DRL=0x14E0C32314DAB389\rdcp 0 spi:DRSS=0xFFFFFFFF00000100\rdcp 0 spi:DRR=0x9D59\rdcp 0 update:u-d\rdcp 0 update:+d\rdcp wait:1h:\rdcp wait::DROVER\rdcp 0 spi:DRL=0x14E60A8714E0C323\rdcp 0 spi:DRSS=0xFFFFFFFF000000D0\rdcp 0 spi:DRR=0x92C9\rdcp 0 update:u-d\rdcp 0 update:+d\rdcp wait:1h:\rdcp wait::DROVER\rdcp 0 spi:DRL=0x14EA8C1314E60A87\rdcp 0 spi:DRSS=0xFFFFFFFF000000A0\rdcp 0 spi:DRR=0x8447\rdcp 0 update:u-d\rdcp 0 update:+d\rdcp wait:1h:\rdcp wait::DROVER\rdcp 0 spi:DRL=0x14EE53ED14EA8C13\rdcp 0 spi:DRSS=0xFFFFFFFF00000004\rdcp 0 spi:DRR=0x3F1\rdcp 0 update:u-d\rdcp 0 update:+d\rdcp wait:1h:\rdcp wait::DROVER\rdcp 0 spi:DRL=0x14F1745114EE53ED\rdcp 0 spi:DRSS=0xFFFFFFFF00000049\rdcp 0 spi:DRR=0x56FB\rdcp 0 update:u-d\rdcp 0 update:+d\rdcp wait:1h:\rdcp wait::DROVER\rdcp 0 spi:DRL=0x14F4025514F17451\rdcp 0 spi:DRSS=0xFFFFFFFF0000008C\rdcp 0 spi:DRR=0xCC25\rdcp 0 update:u-d\rdcp 0 update:+d\rdcp wait:1h:\rdcp wait::DROVER\rdcp 0 spi:DRL=0x14F6138A14F40255\rdcp 0 spi:DRSS=0xFFFFFFFF00000003\rdcp 0 spi:DRR=0x568\rdcp 0 update:u-d\rdcp 0 update:+d\rdcp wait:1h:\rdcp wait::DROVER\rdcp 0 spi:DRL=0x14F7BC5D14F6138A\rdcp 0 spi:DRSS=0xFFFFFFFF00000049\rdcp 0 spi:DRR=0xA3E0\rdcp 0 update:u-d\rdcp 0 update:+d\rdcp wait:1h:\rdcp wait::DROVER\rdcp 0 spi:DRL=0x14F90F3B14F7BC5D\rdcp 0 spi:DRSS=0xFFFFFFFF0000001C\rdcp 0 spi:DRR=0x4ECD\rdcp 0 update:u-d\rdcp 0 update:+d\rdcp wait:1h:\rdcp wait::DROVER\rdcp 0 spi:DRL=0x14FA1C2814F90F3B\rdcp 0 spi:DRSS=0xFFFFFFFF00000006\rdcp 0 spi:DRR=0x1547\rdcp 0 update:u-d\rdcp 0 update:+d\rdcp wait:1h:\rdcp wait::DROVER\rdcp 0 spi:DRL=0x14FAF0B814FA1C28\rdcp 0 spi:DRSS=0xFFFFFFFF0000002B\rdcp 0 spi:DRR=0xC0EC\rdcp 0 update:u-d\rdcp 0 update:+d\rdcp wait:1h:\rdcp wait::DROVER\rdcp 0 spi:DRL=0x14FB983214FAF0B8\rdcp 0 spi:DRSS=0xFFFFFFFF0000000D\rdcp 0 spi:DRR=0x4A07\rdcp 0 update:u-d\rdcp 0 update:+d\rdcp wait:1h:\rdcp wait::DROVER\rdcp 0 spi:DRL=0x14FC1BD114FB9832\rdcp 0 spi:DRSS=0xFFFFFFFF00000009\rdcp 0 spi:DRR=0x4136\rdcp 0 update:u-d\rdcp 0 update:+d\rdcp wait:1h:\rdcp wait::DROVER\rdcp 0 spi:DRL=0x14FC830D14FC1BD1\rdcp 0 spi:DRSS=0xFFFFFFFF00000017\rdcp 0 spi:DRR=0xD478\rdcp 0 update:u-d\rdcp 0 update:+d\rdcp wait:1h:\rdcp wait::DROVER\rdcp 0 spi:DRL=0x14FCD3E614FC830D\rdcp 0 spi:DRSS=0xFFFFFFFF00000004\rdcp 0 spi:DRR=0x2F2F\rdcp 0 update:u-d\rdcp 0 update:+d\rdcp wait:1h:\rdcp wait::DROVER\rdcp 0 spi:DRL=0x14FD132314FCD3E6\rdcp 0 spi:DRSS=0xFFFFFFFF00000003\rdcp 0 spi:DRR=0x2D3E\rdcp 0 update:u-d\rdcp 0 update:+d\rdcp wait:1h:\rdcp wait::DROVER\rdcp 0 spi:DRL=0x14FD448E14FD1323\rdcp 0 spi:DRSS=0xFFFFFFFF00000002\rdcp 0 spi:DRR=0x2699\rdcp 0 update:u-d\rdcp 0 update:+d\rdcp wait:1h:\rdcp wait::DROVER\rdcp start\r"
  out "frequency-time plot":T8(graph)=[{[{"total time[ms]"=0.0, "f1 [Hz] CH0"=80013385.70184857}, {"total time[ms]"=250.0, "f1 [Hz] CH0"=80017154.97082743}, {"total time[ms]"=250.0, "f1 [Hz] CH0"=80017154.97082743}, {"total time[ms]"=500.0, "f1 [Hz] CH0"=80021973.8852612}, {"total time[ms]"=500.0, "f1 [Hz] CH0"=80021973.8852612}, {"total time[ms]"=750.0, "f1 [Hz] CH0"=80028127.2540865}, {"total time[ms]"=750.0, "f1 [Hz] CH0"=80028127.2540865}, {"total time[ms]"=1000.0, "f1 [Hz] CH0"=80035972.41992418}, {"total time[ms]"=1000.0, "f1 [Hz] CH0"=80035972.41992418}, {"total time[ms]"=1250.0, "f1 [Hz] CH0"=80045954.73982005}, {"total time[ms]"=1250.0, "f1 [Hz] CH0"=80045954.73982005}, {"total time[ms]"=1500.0, "f1 [Hz] CH0"=80058624.46150272}, {"total time[ms]"=1500.0, "f1 [Hz] CH0"=80058624.46150272}, {"total time[ms]"=1750.0, "f1 [Hz] CH0"=80074653.77468826}, {"total time[ms]"=1750.0, "f1 [Hz] CH0"=80074653.77468826}, {"total time[ms]"=2000.0, "f1 [Hz] CH0"=80094851.74635513}, {"total time[ms]"=2000.0, "f1 [Hz] CH0"=80094851.74635513}, {"total time[ms]"=2250.0, "f1 [Hz] CH0"=80120173.30034801}, {"total time[ms]"=2250.0, "f1 [Hz] CH0"=80120173.30034801}, {"total time[ms]"=2500.0, "f1 [Hz] CH0"=80151716.36004248}, {"total time[ms]"=2500.0, "f1 [Hz] CH0"=80151716.36004248}, {"total time[ms]"=2750.0, "f1 [Hz] CH0"=80190698.92979822}, {"total time[ms]"=2750.0, "f1 [Hz] CH0"=80190698.92979822}, {"total time[ms]"=3000.0, "f1 [Hz] CH0"=80238405.84404424}, {"total time[ms]"=3000.0, "f1 [Hz] CH0"=80238405.84404424}, {"total time[ms]"=3250.0, "f1 [Hz] CH0"=80296094.39606337}, {"total time[ms]"=3250.0, "f1 [Hz] CH0"=80296094.39606337}, {"total time[ms]"=3500.0, "f1 [Hz] CH0"=80364851.04761271}, {"total time[ms]"=3500.0, "f1 [Hz] CH0"=80364851.04761271}, {"total time[ms]"=3750.0, "f1 [Hz] CH0"=80445400.27765062}, {"total time[ms]"=3750.0, "f1 [Hz] CH0"=80445400.27765062}, {"total time[ms]"=4000.0, "f1 [Hz] CH0"=80537882.84273998}, {"total time[ms]"=4000.0, "f1 [Hz] CH0"=80537882.84273998}, {"total time[ms]"=4250.0, "f1 [Hz] CH0"=80641642.60164921}, {"total time[ms]"=4250.0, "f1 [Hz] CH0"=80641642.60164921}, {"total time[ms]"=4500.0, "f1 [Hz] CH0"=80755081.3375963}, {"total time[ms]"=4500.0, "f1 [Hz] CH0"=80755081.3375963}, {"total time[ms]"=4750.0, "f1 [Hz] CH0"=80875646.9982284}, {"total time[ms]"=4750.0, "f1 [Hz] CH0"=80875646.9982284}, {"total time[ms]"=5000.0, "f1 [Hz] CH0"=81000000.0}, {"total time[ms]"=5000.0, "f1 [Hz] CH0"=81000000.0}, {"total time[ms]"=5250.0, "f1 [Hz] CH0"=81124353.0017716}, {"total time[ms]"=5250.0, "f1 [Hz] CH0"=81124353.0017716}, {"total time[ms]"=5500.0, "f1 [Hz] CH0"=81244918.6624037}, {"total time[ms]"=5500.0, "f1 [Hz] CH0"=81244918.6624037}, {"total time[ms]"=5750.0, "f1 [Hz] CH0"=81358357.39835079}, {"total time[ms]"=5750.0, "f1 [Hz] CH0"=81358357.39835079}, {"total time[ms]"=6000.0, "f1 [Hz] CH0"=81462117.15726002}, {"total time[ms]"=6000.0, "f1 [Hz] CH0"=81462117.15726002}, {"total time[ms]"=6250.0, "f1 [Hz] CH0"=81554599.72234938}, {"total time[ms]"=6250.0, "f1 [Hz] CH0"=81554599.72234938}, {"total time[ms]"=6500.0, "f1 [Hz] CH0"=81635148.95238729}, {"total time[ms]"=6500.0, "f1 [Hz] CH0"=81635148.95238729}, {"total time[ms]"=6750.0, "f1 [Hz] CH0"=81703905.60393663}, {"total time[ms]"=6750.0, "f1 [Hz] CH0"=81703905.60393663}, {"total time[ms]"=7000.0, "f1 [Hz] CH0"=81761594.15595576}, {"total time[ms]"=7000.0, "f1 [Hz] CH0"=81761594.15595576}, {"total time[ms]"=7250.0, "f1 [Hz] CH0"=81809301.07020178}, {"total time[ms]"=7250.0, "f1 [Hz] CH0"=81809301.07020178}, {"total time[ms]"=7500.0, "f1 [Hz] CH0"=81848283.63995752}, {"total time[ms]"=7500.0, "f1 [Hz] CH0"=81848283.63995752}, {"total time[ms]"=7750.0, "f1 [Hz] CH0"=81879826.69965199}, {"total time[ms]"=7750.0, "f1 [Hz] CH0"=81879826.69965199}, {"total time[ms]"=8000.0, "f1 [Hz] CH0"=81905148.25364487}, {"total time[ms]"=8000.0, "f1 [Hz] CH0"=81905148.25364487}, {"total time[ms]"=8250.0, "f1 [Hz] CH0"=81925346.22531174}, {"total time[ms]"=8250.0, "f1 [Hz] CH0"=81925346.22531174}, {"total time[ms]"=8500.0, "f1 [Hz] CH0"=81941375.53849728}, {"total time[ms]"=8500.0, "f1 [Hz] CH0"=81941375.53849728}, {"total time[ms]"=8750.0, "f1 [Hz] CH0"=81954045.26017995}, {"total time[ms]"=8750.0, "f1 [Hz] CH0"=81954045.26017995}, {"total time[ms]"=9000.0, "f1 [Hz] CH0"=81964027.58007582}, {"total time[ms]"=9000.0, "f1 [Hz] CH0"=81964027.58007582}, {"total time[ms]"=9250.0, "f1 [Hz] CH0"=81971872.7459135}, {"total time[ms]"=9250.0, "f1 [Hz] CH0"=81971872.7459135}, {"total time[ms]"=9500.0, "f1 [Hz] CH0"=81978026.1147388}, {"total time[ms]"=9500.0, "f1 [Hz] CH0"=81978026.1147388}, {"total time[ms]"=9750.0, "f1 [Hz] CH0"=81982845.02917257}, {"total time[ms]"=9750.0, "f1 [Hz] CH0"=81982845.02917257}, {"total time[ms]"=10000.0, "f1 [Hz] CH0"=81986614.29815143}, {"total time[ms]"=10000.0, "f1 [Hz] CH0"=81986614.29815143}, {"total time[ms]"=10250.0, "f1 [Hz] CH0"=81989559.74861288}]}, {[{"total time[ms]"=0.0, "f1 [Hz] CH0"=80000000.0}, {"total time[ms]"=250.0, "f1 [Hz] CH0"=80000000.0}, {"total time[ms]"=250.0, "f1 [Hz] CH0"=80000000.0}, {"total time[ms]"=500.0, "f1 [Hz] CH0"=80000000.0}, {"total time[ms]"=500.0, "f1 [Hz] CH0"=80000000.0}, {"total time[ms]"=750.0, "f1 [Hz] CH0"=80000000.0}, {"total time[ms]"=750.0, "f1 [Hz] CH0"=80000000.0}, {"total time[ms]"=1000.0, "f1 [Hz] CH0"=80000000.0}, {"total time[ms]"=1000.0, "f1 [Hz] CH0"=80000000.0}, {"total time[ms]"=1250.0, "f1 [Hz] CH0"=80000000.0}, {"total time[ms]"=1250.0, "f1 [Hz] CH0"=80000000.0}, {"total time[ms]"=1500.0, "f1 [Hz] CH0"=80000000.0}, {"total time[ms]"=1500.0, "f1 [Hz] CH0"=80000000.0}, {"total time[ms]"=1750.0, "f1 [Hz] CH0"=80000000.0}, {"total time[ms]"=1750.0, "f1 [Hz] CH0"=80000000.0}, {"total time[ms]"=2000.0, "f1 [Hz] CH0"=80000000.0}, {"total time[ms]"=2000.0, "f1 [Hz] CH0"=80000000.0}, {"total time[ms]"=2250.0, "f1 [Hz] CH0"=80000000.0}, {"total time[ms]"=2250.0, "f1 [Hz] CH0"=80000000.0}, {"total time[ms]"=2500.0, "f1 [Hz] CH0"=80000000.0}, {"total time[ms]"=2500.0, "f1 [Hz] CH0"=80000000.0}, {"total time[ms]"=2750.0, "f1 [Hz] CH0"=80000000.0}, {"total time[ms]"=2750.0, "f1 [Hz] CH0"=80000000.0}, {"total time[ms]"=3000.0, "f1 [Hz] CH0"=80000000.0}, {"total time[ms]"=3000.0, "f1 [Hz] CH0"=80000000.0}, {"total time[ms]"=3250.0, "f1 [Hz] CH0"=80000000.0}, {"total time[ms]"=3250.0, "f1 [Hz] CH0"=80000000.0}, {"total time[ms]"=3500.0, "f1 [Hz] CH0"=80000000.0}, {"total time[ms]"=3500.0, "f1 [Hz] CH0"=80000000.0}, {"total time[ms]"=3750.0, "f1 [Hz] CH0"=80000000.0}, {"total time[ms]"=3750.0, "f1 [Hz] CH0"=80000000.0}, {"total time[ms]"=4000.0, "f1 [Hz] CH0"=80000000.0}, {"total time[ms]"=4000.0, "f1 [Hz] CH0"=80000000.0}, {"total time[ms]"=4250.0, "f1 [Hz] CH0"=80000000.0}, {"total time[ms]"=4250.0, "f1 [Hz] CH0"=80000000.0}, {"total time[ms]"=4500.0, "f1 [Hz] CH0"=80000000.0}, {"total time[ms]"=4500.0, "f1 [Hz] CH0"=80000000.0}, {"total time[ms]"=4750.0, "f1 [Hz] CH0"=80000000.0}, {"total time[ms]"=4750.0, "f1 [Hz] CH0"=80000000.0}, {"total time[ms]"=5000.0, "f1 [Hz] CH0"=80000000.0}, {"total time[ms]"=5000.0, "f1 [Hz] CH0"=80000000.0}, {"total time[ms]"=5250.0, "f1 [Hz] CH0"=80000000.0}, {"total time[ms]"=5250.0, "f1 [Hz] CH0"=80000000.0}, {"total time[ms]"=5500.0, "f1 [Hz] CH0"=80000000.0}, {"total time[ms]"=5500.0, "f1 [Hz] CH0"=80000000.0}, {"total time[ms]"=5750.0, "f1 [Hz] CH0"=80000000.0}, {"total time[ms]"=5750.0, "f1 [Hz] CH0"=80000000.0}, {"total time[ms]"=6000.0, "f1 [Hz] CH0"=80000000.0}, {"total time[ms]"=6000.0, "f1 [Hz] CH0"=80000000.0}, {"total time[ms]"=6250.0, "f1 [Hz] CH0"=80000000.0}, {"total time[ms]"=6250.0, "f1 [Hz] CH0"=80000000.0}, {"total time[ms]"=6500.0, "f1 [Hz] CH0"=80000000.0}, {"total time[ms]"=6500.0, "f1 [Hz] CH0"=80000000.0}, {"total time[ms]"=6750.0, "f1 [Hz] CH0"=80000000.0}, {"total time[ms]"=6750.0, "f1 [Hz] CH0"=80000000.0}, {"total time[ms]"=7000.0, "f1 [Hz] CH0"=80000000.0}, {"total time[ms]"=7000.0, "f1 [Hz] CH0"=80000000.0}, {"total time[ms]"=7250.0, "f1 [Hz] CH0"=80000000.0}, {"total time[ms]"=7250.0, "f1 [Hz] CH0"=80000000.0}, {"total time[ms]"=7500.0, "f1 [Hz] CH0"=80000000.0}, {"total time[ms]"=7500.0, "f1 [Hz] CH0"=80000000.0}, {"total time[ms]"=7750.0, "f1 [Hz] CH0"=80000000.0}, {"total time[ms]"=7750.0, "f1 [Hz] CH0"=80000000.0}, {"total time[ms]"=8000.0, "f1 [Hz] CH0"=80000000.0}, {"total time[ms]"=8000.0, "f1 [Hz] CH0"=80000000.0}, {"total time[ms]"=8250.0, "f1 [Hz] CH0"=80000000.0}, {"total time[ms]"=8250.0, "f1 [Hz] CH0"=80000000.0}, {"total time[ms]"=8500.0, "f1 [Hz] CH0"=80000000.0}, {"total time[ms]"=8500.0, "f1 [Hz] CH0"=80000000.0}, {"total time[ms]"=8750.0, "f1 [Hz] CH0"=80000000.0}, {"total time[ms]"=8750.0, "f1 [Hz] CH0"=80000000.0}, {"total time[ms]"=9000.0, "f1 [Hz] CH0"=80000000.0}, {"total time[ms]"=9000.0, "f1 [Hz] CH0"=80000000.0}, {"total time[ms]"=9250.0, "f1 [Hz] CH0"=80000000.0}, {"total time[ms]"=9250.0, "f1 [Hz] CH0"=80000000.0}, {"total time[ms]"=9500.0, "f1 [Hz] CH0"=80000000.0}, {"total time[ms]"=9500.0, "f1 [Hz] CH0"=80000000.0}, {"total time[ms]"=9750.0, "f1 [Hz] CH0"=80000000.0}, {"total time[ms]"=9750.0, "f1 [Hz] CH0"=80000000.0}, {"total time[ms]"=10000.0, "f1 [Hz] CH0"=80000000.0}, {"total time[ms]"=10000.0, "f1 [Hz] CH0"=80000000.0}, {"total time[ms]"=10250.0, "f1 [Hz] CH0"=80000000.0}]}]
  in  "Control Elements Array":T9(array[cluster])=[{"STEP"=0, "time[ms]"=250.0, "time tolerance[us]"=0.01, "CH0"=TRUE, "rel. amplitude CH0"=1.0, "phase [°] CH0"=0.0, "f0 [Hz] CH0"=80013385.70184857, "f1 [Hz] CH0"=80017154.97082743, "CH1"=TRUE, "rel. amplitude CH1"=1.0, "phase [°] CH1"=0.0, "f0 [Hz] CH1"=80000000.0, "f1 [Hz] CH1"=80000000.0}, {"STEP"=0, "time[ms]"=250.0, "time tolerance[us]"=0.01, "CH0"=TRUE, "rel. amplitude CH0"=1.0, "phase [°] CH0"=0.0, "f0 [Hz] CH0"=80017154.97082743, "f1 [Hz] CH0"=80021973.8852612, "CH1"=FALSE, "rel. amplitude CH1"=1.0, "phase [°] CH1"=0.0, "f0 [Hz] CH1"=80000000.0, "f1 [Hz] CH1"=80000000.0}, {"STEP"=0, "time[ms]"=250.0, "time tolerance[us]"=0.01, "CH0"=TRUE, "rel. amplitude CH0"=1.0, "phase [°] CH0"=0.0, "f0 [Hz] CH0"=80021973.8852612, "f1 [Hz] CH0"=80028127.2540865, "CH1"=FALSE, "rel. amplitude CH1"=1.0, "phase [°] CH1"=0.0, "f0 [Hz] CH1"=80000000.0, "f1 [Hz] CH1"=80000000.0}, {"STEP"=0, "time[ms]"=250.0, "time tolerance[us]"=0.01, "CH0"=TRUE, "rel. amplitude CH0"=1.0, "phase [°] CH0"=0.0, "f0 [Hz] CH0"=80028127.2540865, "f1 [Hz] CH0"=80035972.41992418, "CH1"=FALSE, "rel. amplitude CH1"=1.0, "phase [°] CH1"=0.0, "f0 [Hz] CH1"=80000000.0, "f1 [Hz] CH1"=80000000.0}, {"STEP"=0, "time[ms]"=250.0, "time tolerance[us]"=0.01, "CH0"=TRUE, "rel. amplitude CH0"=1.0, "phase [°] CH0"=0.0, "f0 [Hz] CH0"=80035972.41992418, "f1 [Hz] CH0"=80045954.73982005, "CH1"=FALSE, "rel. amplitude CH1"=1.0, "phase [°] CH1"=0.0, "f0 [Hz] CH1"=80000000.0, "f1 [Hz] CH1"=80000000.0}, {"STEP"=0, "time[ms]"=250.0, "time tolerance[us]"=0.01, "CH0"=TRUE, "rel. amplitude CH0"=1.0, "phase [°] CH0"=0.0, "f0 [Hz] CH0"=80045954.73982005, "f1 [Hz] CH0"=80058624.46150272, "CH1"=FALSE, "rel. amplitude CH1"=1.0, "phase [°] CH1"=0.0, "f0 [Hz] CH1"=80000000.0, "f1 [Hz] CH1"=80000000.0}, {"STEP"=0, "time[ms]"=250.0, "time tolerance[us]"=0.01, "CH0"=TRUE, "rel. amplitude CH0"=1.0, "phase [°] CH0"=0.0, "f0 [Hz] CH0"=80058624.46150272, "f1 [Hz] CH0"=80074653.77468826, "CH1"=FALSE, "rel. amplitude CH1"=1.0, "phase [°] CH1"=0.0, "f0 [Hz] CH1"=80000000.0, "f1 [Hz] CH1"=80000000.0}, {"STEP"=0, "time[ms]"=250.0, "time tolerance[us]"=0.01, "CH0"=TRUE, "rel. amplitude CH0"=1.0, "phase [°] CH0"=0.0, "f0 [Hz] CH0"=80074653.77468826, "f1 [Hz] CH0"=80094851.74635513, "CH1"=FALSE, "rel. amplitude CH1"=1.0, "phase [°] CH1"=0.0, "f0 [Hz] CH1"=80000000.0, "f1 [Hz] CH1"=80000000.0}, {"STEP"=0, "time[ms]"=250.0, "time tolerance[us]"=0.01, "CH0"=TRUE, "rel. amplitude CH0"=1.0, "phase [°] CH0"=0.0, "f0 [Hz] CH0"=80094851.74635513, "f1 [Hz] CH0"=80120173.30034801, "CH1"=FALSE, "rel. amplitude CH1"=1.0, "phase [°] CH1"=0.0, "f0 [Hz] CH1"=80000000.0, "f1 [Hz] CH1"=80000000.0}, {"STEP"=0, "time[ms]"=250.0, "time tolerance[us]"=0.01, "CH0"=TRUE, "rel. amplitude CH0"=1.0, "phase [°] CH0"=0.0, "f0 [Hz] CH0"=80120173.30034801, "f1 [Hz] CH0"=80151716.36004248, "CH1"=FALSE, "rel. amplitude CH1"=1.0, "phase [°] CH1"=0.0, "f0 [Hz] CH1"=80000000.0, "f1 [Hz] CH1"=80000000.0}, {"STEP"=0, "time[ms]"=250.0, "time tolerance[us]"=0.01, "CH0"=TRUE, "rel. amplitude CH0"=1.0, "phase [°] CH0"=0.0, "f0 [Hz] CH0"=80151716.36004248, "f1 [Hz] CH0"=80190698.92979822, "CH1"=FALSE, "rel. amplitude CH1"=1.0, "phase [°] CH1"=0.0, "f0 [Hz] CH1"=80000000.0, "f1 [Hz] CH1"=80000000.0}, {"STEP"=0, "time[ms]"=250.0, "time tolerance[us]"=0.01, "CH0"=TRUE, "rel. amplitude CH0"=1.0, "phase [°] CH0"=0.0, "f0 [Hz] CH0"=80190698.92979822, "f1 [Hz] CH0"=80238405.84404424, "CH1"=FALSE, "rel. amplitude CH1"=1.0, "phase [°] CH1"=0.0, "f0 [Hz] CH1"=80000000.0, "f1 [Hz] CH1"=80000000.0}, {"STEP"=0, "time[ms]"=250.0, "time tolerance[us]"=0.01, "CH0"=TRUE, "rel. amplitude CH0"=1.0, "phase [°] CH0"=0.0, "f0 [Hz] CH0"=80238405.84404424, "f1 [Hz] CH0"=80296094.39606337, "CH1"=FALSE, "rel. amplitude CH1"=1.0, "phase [°] CH1"=0.0, "f0 [Hz] CH1"=80000000.0, "f1 [Hz] CH1"=80000000.0}, {"STEP"=0, "time[ms]"=250.0, "time tolerance[us]"=0.01, "CH0"=TRUE, "rel. amplitude CH0"=1.0, "phase [°] CH0"=0.0, "f0 [Hz] CH0"=80296094.39606337, "f1 [Hz] CH0"=80364851.04761271, "CH1"=FALSE, "rel. amplitude CH1"=1.0, "phase [°] CH1"=0.0, "f0 [Hz] CH1"=80000000.0, "f1 [Hz] CH1"=80000000.0}, {"STEP"=0, "time[ms]"=250.0, "time tolerance[us]"=0.01, "CH0"=TRUE, "rel. amplitude CH0"=1.0, "phase [°] CH0"=0.0, "f0 [Hz] CH0"=80364851.04761271, "f1 [Hz] CH0"=80445400.27765062, "CH1"=FALSE, "rel. amplitude CH1"=1.0, "phase [°] CH1"=0.0, "f0 [Hz] CH1"=80000000.0, "f1 [Hz] CH1"=80000000.0}, {"STEP"=0, "time[ms]"=250.0, "time tolerance[us]"=0.01, "CH0"=TRUE, "rel. amplitude CH0"=1.0, "phase [°] CH0"=0.0, "f0 [Hz] CH0"=80445400.27765062, "f1 [Hz] CH0"=80537882.84273998, "CH1"=FALSE, "rel. amplitude CH1"=1.0, "phase [°] CH1"=0.0, "f0 [Hz] CH1"=80000000.0, "f1 [Hz] CH1"=80000000.0}, {"STEP"=0, "time[ms]"=250.0, "time tolerance[us]"=0.01, "CH0"=TRUE, "rel. amplitude CH0"=1.0, "phase [°] CH0"=0.0, "f0 [Hz] CH0"=80537882.84273998, "f1 [Hz] CH0"=80641642.60164921, "CH1"=FALSE, "rel. amplitude CH1"=1.0, "phase [°] CH1"=0.0, "f0 [Hz] CH1"=80000000.0, "f1 [Hz] CH1"=80000000.0}, {"STEP"=0, "time[ms]"=250.0, "time tolerance[us]"=0.01, "CH0"=TRUE, "rel. amplitude CH0"=1.0, "phase [°] CH0"=0.0, "f0 [Hz] CH0"=80641642.60164921, "f1 [Hz] CH0"=80755081.3375963, "CH1"=FALSE, "rel. amplitude CH1"=1.0, "phase [°] CH1"=0.0, "f0 [Hz] CH1"=80000000.0, "f1 [Hz] CH1"=80000000.0}, {"STEP"=0, "time[ms]"=250.0, "time tolerance[us]"=0.01, "CH0"=TRUE, "rel. amplitude CH0"=1.0, "phase [°] CH0"=0.0, "f0 [Hz] CH0"=80755081.3375963, "f1 [Hz] CH0"=80875646.9982284, "CH1"=FALSE, "rel. amplitude CH1"=1.0, "phase [°] CH1"=0.0, "f0 [Hz] CH1"=80000000.0, "f1 [Hz] CH1"=80000000.0}, {"STEP"=0, "time[ms]"=250.0, "time tolerance[us]"=0.01, "CH0"=TRUE, "rel. amplitude CH0"=1.0, "phase [°] CH0"=0.0, "f0 [Hz] CH0"=80875646.9982284, "f1 [Hz] CH0"=81000000.0, "CH1"=FALSE, "rel. amplitude CH1"=1.0, "phase [°] CH1"=0.0, "f0 [Hz] CH1"=80000000.0, "f1 [Hz] CH1"=80000000.0}, {"STEP"=0, "time[ms]"=250.0, "time tolerance[us]"=0.01, "CH0"=TRUE, "rel. amplitude CH0"=1.0, "phase [°] CH0"=0.0, "f0 [Hz] CH0"=81000000.0, "f1 [Hz] CH0"=81124353.0017716, "CH1"=FALSE, "rel. amplitude CH1"=1.0, "phase [°] CH1"=0.0, "f0 [Hz] CH1"=80000000.0, "f1 [Hz] CH1"=80000000.0}, {"STEP"=0, "time[ms]"=250.0, "time tolerance[us]"=0.01, "CH0"=TRUE, "rel. amplitude CH0"=1.0, "phase [°] CH0"=0.0, "f0 [Hz] CH0"=81124353.0017716, "f1 [Hz] CH0"=81244918.6624037, "CH1"=FALSE, "rel. amplitude CH1"=1.0, "phase [°] CH1"=0.0, "f0 [Hz] CH1"=80000000.0, "f1 [Hz] CH1"=80000000.0}, {"STEP"=0, "time[ms]"=250.0, "time tolerance[us]"=0.01, "CH0"=TRUE, "rel. amplitude CH0"=1.0, "phase [°] CH0"=0.0, "f0 [Hz] CH0"=81244918.6624037, "f1 [Hz] CH0"=81358357.39835079, "CH1"=FALSE, "rel. amplitude CH1"=1.0, "phase [°] CH1"=0.0, "f0 [Hz] CH1"=80000000.0, "f1 [Hz] CH1"=80000000.0}, {"STEP"=0, "time[ms]"=250.0, "time tolerance[us]"=0.01, "CH0"=TRUE, "rel. amplitude CH0"=1.0, "phase [°] CH0"=0.0, "f0 [Hz] CH0"=81358357.39835079, "f1 [Hz] CH0"=81462117.15726002, "CH1"=FALSE, "rel. amplitude CH1"=1.0, "phase [°] CH1"=0.0, "f0 [Hz] CH1"=80000000.0, "f1 [Hz] CH1"=80000000.0}, {"STEP"=0, "time[ms]"=250.0, "time tolerance[us]"=0.01, "CH0"=TRUE, "rel. amplitude CH0"=1.0, "phase [°] CH0"=0.0, "f0 [Hz] CH0"=81462117.15726002, "f1 [Hz] CH0"=81554599.72234938, "CH1"=FALSE, "rel. amplitude CH1"=1.0, "phase [°] CH1"=0.0, "f0 [Hz] CH1"=80000000.0, "f1 [Hz] CH1"=80000000.0}, {"STEP"=0, "time[ms]"=250.0, "time tolerance[us]"=0.01, "CH0"=TRUE, "rel. amplitude CH0"=1.0, "phase [°] CH0"=0.0, "f0 [Hz] CH0"=81554599.72234938, "f1 [Hz] CH0"=81635148.95238729, "CH1"=FALSE, "rel. amplitude CH1"=1.0, "phase [°] CH1"=0.0, "f0 [Hz] CH1"=80000000.0, "f1 [Hz] CH1"=80000000.0}, {"STEP"=0, "time[ms]"=250.0, "time tolerance[us]"=0.01, "CH0"=TRUE, "rel. amplitude CH0"=1.0, "phase [°] CH0"=0.0, "f0 [Hz] CH0"=81635148.95238729, "f1 [Hz] CH0"=81703905.60393663, "CH1"=FALSE, "rel. amplitude CH1"=1.0, "phase [°] CH1"=0.0, "f0 [Hz] CH1"=80000000.0, "f1 [Hz] CH1"=80000000.0}, {"STEP"=0, "time[ms]"=250.0, "time tolerance[us]"=0.01, "CH0"=TRUE, "rel. amplitude CH0"=1.0, "phase [°] CH0"=0.0, "f0 [Hz] CH0"=81703905.60393663, "f1 [Hz] CH0"=81761594.15595576, "CH1"=FALSE, "rel. amplitude CH1"=1.0, "phase [°] CH1"=0.0, "f0 [Hz] CH1"=80000000.0, "f1 [Hz] CH1"=80000000.0}, {"STEP"=0, "time[ms]"=250.0, "time tolerance[us]"=0.01, "CH0"=TRUE, "rel. amplitude CH0"=1.0, "phase [°] CH0"=0.0, "f0 [Hz] CH0"=81761594.15595576, "f1 [Hz] CH0"=81809301.07020178, "CH1"=FALSE, "rel. amplitude CH1"=1.0, "phase [°] CH1"=0.0, "f0 [Hz] CH1"=80000000.0, "f1 [Hz] CH1"=80000000.0}, {"STEP"=0, "time[ms]"=250.0, "time tolerance[us]"=0.01, "CH0"=TRUE, "rel. amplitude CH0"=1.0, "phase [°] CH0"=0.0, "f0 [Hz] CH0"=81809301.07020178, "f1 [Hz] CH0"=81848283.63995752, "CH1"=FALSE, "rel. amplitude CH1"=1.0, "phase [°] CH1"=0.0, "f0 [Hz] CH1"=80000000.0, "f1 [Hz] CH1"=80000000.0}, {"STEP"=0, "time[ms]"=250.0, "time tolerance[us]"=0.01, "CH0"=TRUE, "rel. amplitude CH0"=1.0, "phase [°] CH0"=0.0, "f0 [Hz] CH0"=81848283.63995752, "f1 [Hz] CH0"=81879826.69965199, "CH1"=FALSE, "rel. amplitude CH1"=1.0, "phase [°] CH1"=0.0, "f0 [Hz] CH1"=80000000.0, "f1 [Hz] CH1"=80000000.0}, {"STEP"=0, "time[ms]"=250.0, "time tolerance[us]"=0.01, "CH0"=TRUE, "rel. amplitude CH0"=1.0, "phase [°] CH0"=0.0, "f0 [Hz] CH0"=81879826.69965199, "f1 [Hz] CH0"=81905148.25364487, "CH1"=FALSE, "rel. amplitude CH1"=1.0, "phase [°] CH1"=0.0, "f0 [Hz] CH1"=80000000.0, "f1 [Hz] CH1"=80000000.0}, {"STEP"=0, "time[ms]"=250.0, "time tolerance[us]"=0.01, "CH0"=TRUE, "rel. amplitude CH0"=1.0, "phase [°] CH0"=0.0, "f0 [Hz] CH0"=81905148.25364487, "f1 [Hz] CH0"=81925346.22531174, "CH1"=FALSE, "rel. amplitude CH1"=1.0, "phase [°] CH1"=0.0, "f0 [Hz] CH1"=80000000.0, "f1 [Hz] CH1"=80000000.0}, {"STEP"=0, "time[ms]"=250.0, "time tolerance[us]"=0.01, "CH0"=TRUE, "rel. amplitude CH0"=1.0, "phase [°] CH0"=0.0, "f0 [Hz] CH0"=81925346.22531174, "f1 [Hz] CH0"=81941375.53849728, "CH1"=FALSE, "rel. amplitude CH1"=1.0, "phase [°] CH1"=0.0, "f0 [Hz] CH1"=80000000.0, "f1 [Hz] CH1"=80000000.0}, {"STEP"=0, "time[ms]"=250.0, "time tolerance[us]"=0.01, "CH0"=TRUE, "rel. amplitude CH0"=1.0, "phase [°] CH0"=0.0, "f0 [Hz] CH0"=81941375.53849728, "f1 [Hz] CH0"=81954045.26017995, "CH1"=FALSE, "rel. amplitude CH1"=1.0, "phase [°] CH1"=0.0, "f0 [Hz] CH1"=80000000.0, "f1 [Hz] CH1"=80000000.0}, {"STEP"=0, "time[ms]"=250.0, "time tolerance[us]"=0.01, "CH0"=TRUE, "rel. amplitude CH0"=1.0, "phase [°] CH0"=0.0, "f0 [Hz] CH0"=81954045.26017995, "f1 [Hz] CH0"=81964027.58007582, "CH1"=FALSE, "rel. amplitude CH1"=1.0, "phase [°] CH1"=0.0, "f0 [Hz] CH1"=80000000.0, "f1 [Hz] CH1"=80000000.0}, {"STEP"=0, "time[ms]"=250.0, "time tolerance[us]"=0.01, "CH0"=TRUE, "rel. amplitude CH0"=1.0, "phase [°] CH0"=0.0, "f0 [Hz] CH0"=81964027.58007582, "f1 [Hz] CH0"=81971872.7459135, "CH1"=FALSE, "rel. amplitude CH1"=1.0, "phase [°] CH1"=0.0, "f0 [Hz] CH1"=80000000.0, "f1 [Hz] CH1"=80000000.0}, {"STEP"=0, "time[ms]"=250.0, "time tolerance[us]"=0.01, "CH0"=TRUE, "rel. amplitude CH0"=1.0, "phase [°] CH0"=0.0, "f0 [Hz] CH0"=81971872.7459135, "f1 [Hz] CH0"=81978026.1147388, "CH1"=FALSE, "rel. amplitude CH1"=1.0, "phase [°] CH1"=0.0, "f0 [Hz] CH1"=80000000.0, "f1 [Hz] CH1"=80000000.0}, {"STEP"=0, "time[ms]"=250.0, "time tolerance[us]"=0.01, "CH0"=TRUE, "rel. amplitude CH0"=1.0, "phase [°] CH0"=0.0, "f0 [Hz] CH0"=81978026.1147388, "f1 [Hz] CH0"=81982845.02917257, "CH1"=FALSE, "rel. amplitude CH1"=1.0, "phase [°] CH1"=0.0, "f0 [Hz] CH1"=80000000.0, "f1 [Hz] CH1"=80000000.0}, {"STEP"=0, "time[ms]"=250.0, "time tolerance[us]"=0.01, "CH0"=TRUE, "rel. amplitude CH0"=1.0, "phase [°] CH0"=0.0, "f0 [Hz] CH0"=81982845.02917257, "f1 [Hz] CH0"=81986614.29815143, "CH1"=FALSE, "rel. amplitude CH1"=1.0, "phase [°] CH1"=0.0, "f0 [Hz] CH1"=80000000.0, "f1 [Hz] CH1"=80000000.0}, {"STEP"=0, "time[ms]"=250.0, "time tolerance[us]"=0.01, "CH0"=TRUE, "rel. amplitude CH0"=1.0, "phase [°] CH0"=0.0, "f0 [Hz] CH0"=81986614.29815143, "f1 [Hz] CH0"=81989559.74861288, "CH1"=FALSE, "rel. amplitude CH1"=1.0, "phase [°] CH1"=0.0, "f0 [Hz] CH1"=80000000.0, "f1 [Hz] CH1"=80000000.0}]
  out "error out":errorcluster={"status"=TRUE, "code"=-1073807339, "source"="VISA Read in FlexDDS-NG_USB_Example.vi"}
  out "read buffer":string
  in  "FlexDDS-NG USB VISA resource name (COM)":refnum<visa-resource-name>="COM5"
  # "STEP"
  # "time [ms]"
  # "time tolerance [us]"
  # "CH0 [false=wait, keep phase&amplitude]"
  # "rel. amplitude CH0"
  # "phase [°] CH0"
  # "f0 [Hz] CH0"
  # "f1 [Hz] CH0"
  # "CH1 [false=wait, keep phase&amplitude]"
  # "rel. amplitude CH1"
  # "phase [°] CH1"
  # "f0 [Hz] CH1"
  # "f1 [Hz] CH1"
  # "f(t) = f0 + (f1-f0)/(1+exp(-k/Dt * (t-Dt/2)))"
  # "f(t) = f1 - (f1-f0)*exp(-K*t/Dt)"
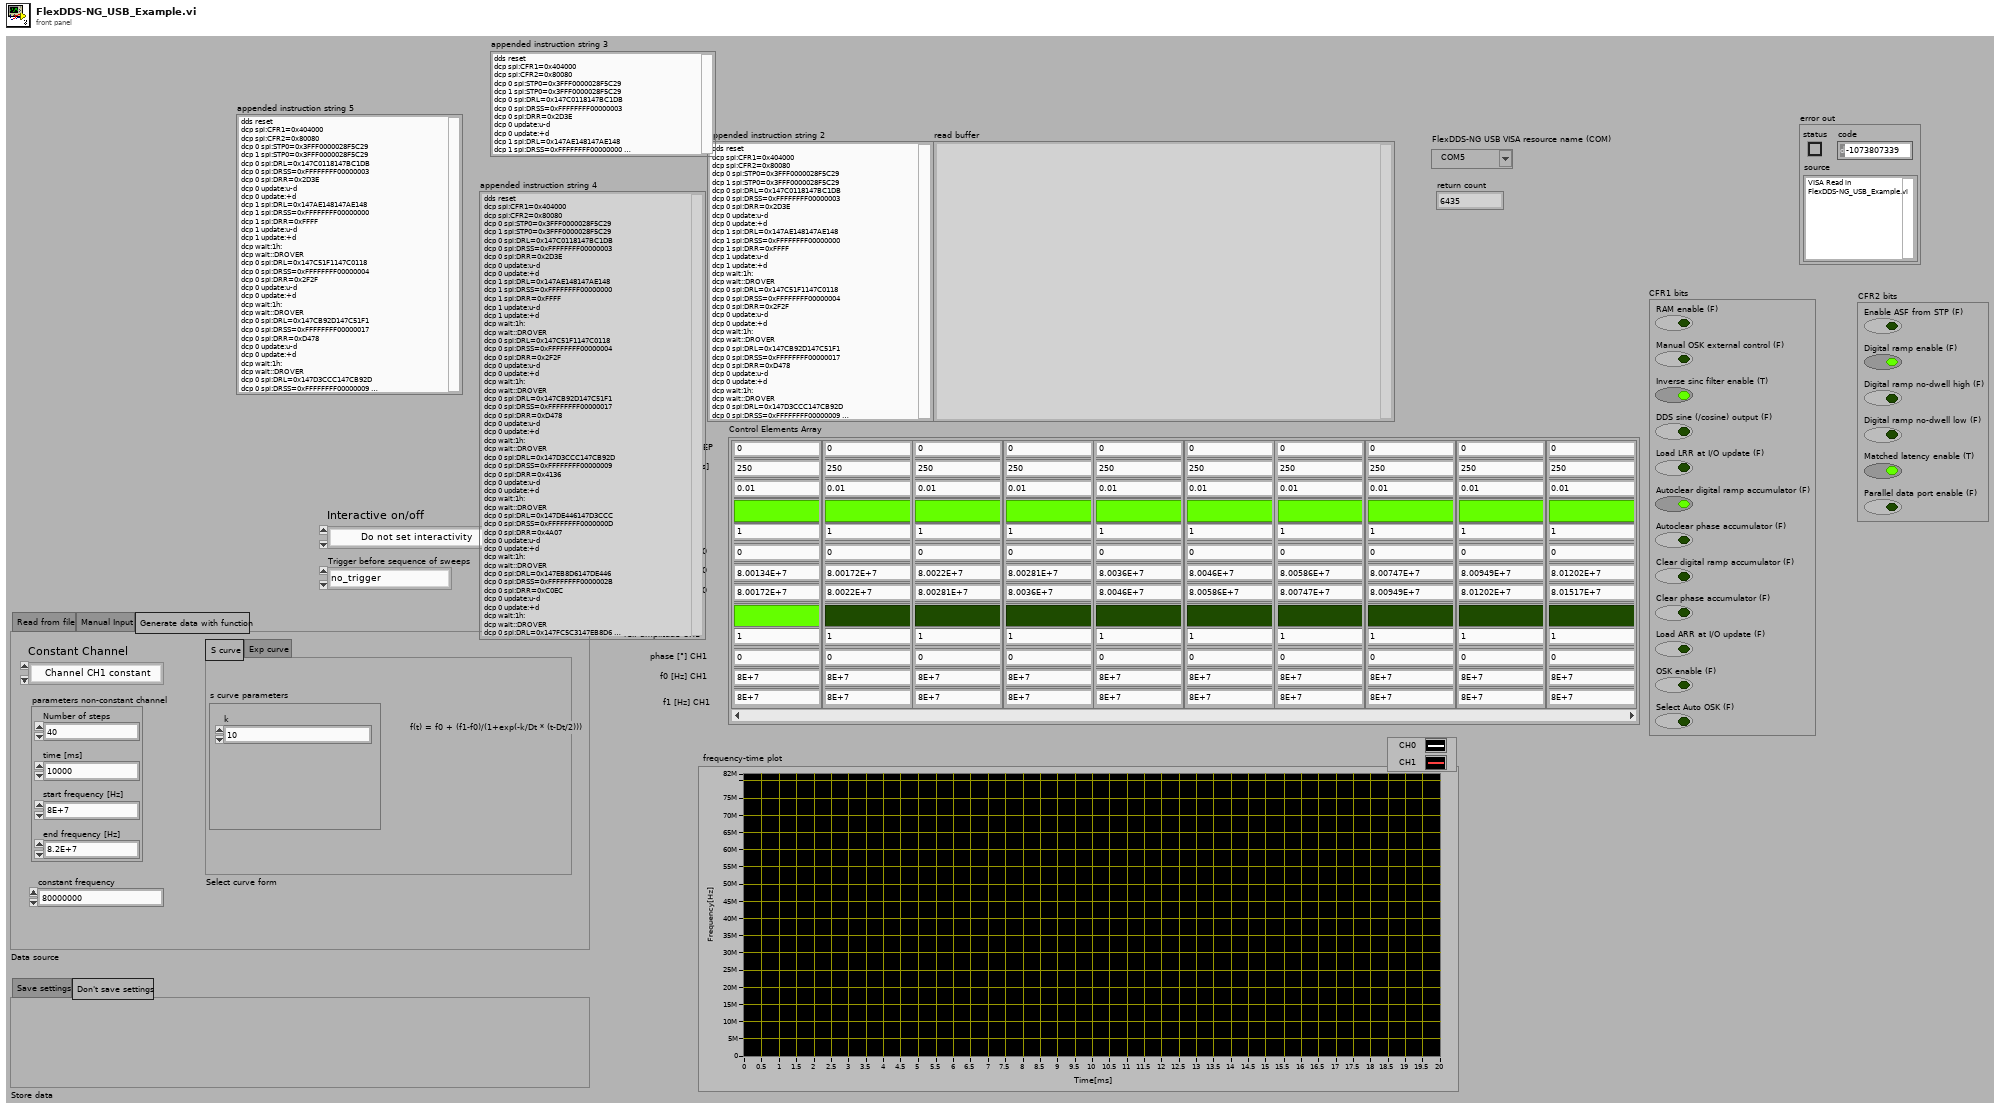
[diagram p1: front panel]
types:
  T1 = enum16{"Do not set interactivity", "Interactive off", "Interactive on"}
  T2 = enum32{"Read from file", "Manual Input", "Generate data with function"}
  T3 = cluster{"Number of steps":i32, "time [ms]":dbl, "start frequency [Hz]":dbl, "end frequency [Hz]":dbl}
  T4 = enum16{"Channel CH1 constant", "Channel CH0 constant"}
  T5 = cluster{"Enable ASF from STP (F)":bool, "Digital ramp enable (F)":bool, "Digital ramp no-dwell high (F)":bool, "Digital ramp no-dwell low (F)":bool, "Matched latency enable (T)":bool, "Parallel data port enable (F)":bool}
  T6 = cluster{"RAM enable (F)":bool, "Manual OSK external control (F)":bool, "Inverse sinc filter enable (T)":bool, "DDS sine (/cosine) output (F)":bool, "Load LRR at I/O update (F)":bool, "Autoclear digital ramp accumulator (F)":bool, "Autoclear phase accumulator (F)":bool, "Clear digital ramp accumulator (F)":bool, "Clear phase accumulator (F)":bool, "Load ARR at I/O update (F)":bool, "OSK enable (F)":bool, "Select Auto OSK (F)":bool}
  T7 = enum16{"no_trigger", "BNC_IN_A_RISING", "BNC_IN_A_FALLING", "BNC_IN_B_RISING", "BNC_IN_B_FALLING", "BNC_IN_C_RISING", "BNC_IN_C_FALLING"}
  T8 = cluster{cluster{"total time[ms]":dbl, "f1 [Hz] CH0":dbl}[]}[]
  T9 = cluster{"STEP":i32, "time[ms]":dbl, "time tolerance[us]":dbl, "CH0":bool, "rel. amplitude CH0":dbl, "phase [°] CH0":dbl, "f0 [Hz] CH0":dbl, "f1 [Hz] CH0":dbl, "CH1":bool, "rel. amplitude CH1":dbl, "phase [°] CH1":dbl, "f0 [Hz] CH1":dbl, "f1 [Hz] CH1":dbl}[]
  T10 = cluster{i32, dbl, "time tolerance":dbl, bool, dbl, dbl, "constant frequency":dbl, "constant frequency":dbl, bool, dbl, dbl, "constant frequency":dbl, "constant frequency":dbl}[]
  T11 = cluster{i32, dbl, "time tolerance":dbl, bool, dbl, dbl, "constant frequency":dbl, "constant frequency":dbl, bool, dbl, dbl, "constant frequency":dbl, "constant frequency":dbl}
  T12 = cluster{"total time[ms]":dbl, "f1 [Hz] CH1":dbl}[]
  T13 = cluster{"total time[ms]":dbl, "f1 [Hz] CH0":dbl}[]
  T14 = cluster{"STEP":i32, "time[ms]":dbl, "time tolerance[us]":dbl, "CH0":bool, "rel. amplitude CH0":dbl, "phase [°] CH0":dbl, "f0 [Hz] CH0":dbl, "f1 [Hz] CH0":dbl, "CH1":bool, "rel. amplitude CH1":dbl, "phase [°] CH1":dbl, "f0 [Hz] CH1":dbl, "f1 [Hz] CH1":dbl}
  T15 = cluster{"Array":cluster{"total time[ms]":dbl, "f1 [Hz] CH0":dbl}[]}
  T16 = cluster{"Array":cluster{"total time[ms]":dbl, "f1 [Hz] CH1":dbl}[]}
  T17 = cluster{"Array":cluster{"total time[ms]":dbl, "f1 [Hz] CH1":dbl}[]}[]
  T18 = enum32{"Channel 0", "Channel 1", "Both channels"}
  T19 = enum32{"O_RAMP_SWP_OVR", "RAM_SWP_OVR", "O_DROVER", "DROVER", "O_SPI_FIFO_EV1", "SPI_FIFO_EV1", "O_SPI_FIFO_EV0", "SPI_FIFO_EV0", "O_SPI_FIFO_FLUSHED", "SPI_FIFO_FLUSHED", "BNC_IN_B_LEVEL", "BNC_IN_B_FALLING", "BNC_IN_B_RISING", "BNC_IN_A_LEVEL", "BNC_IN_A_FALLING", "BNC_IN_A_RISING", "ALL_SPI_FIFOS_FLUSHED", "NONE"}
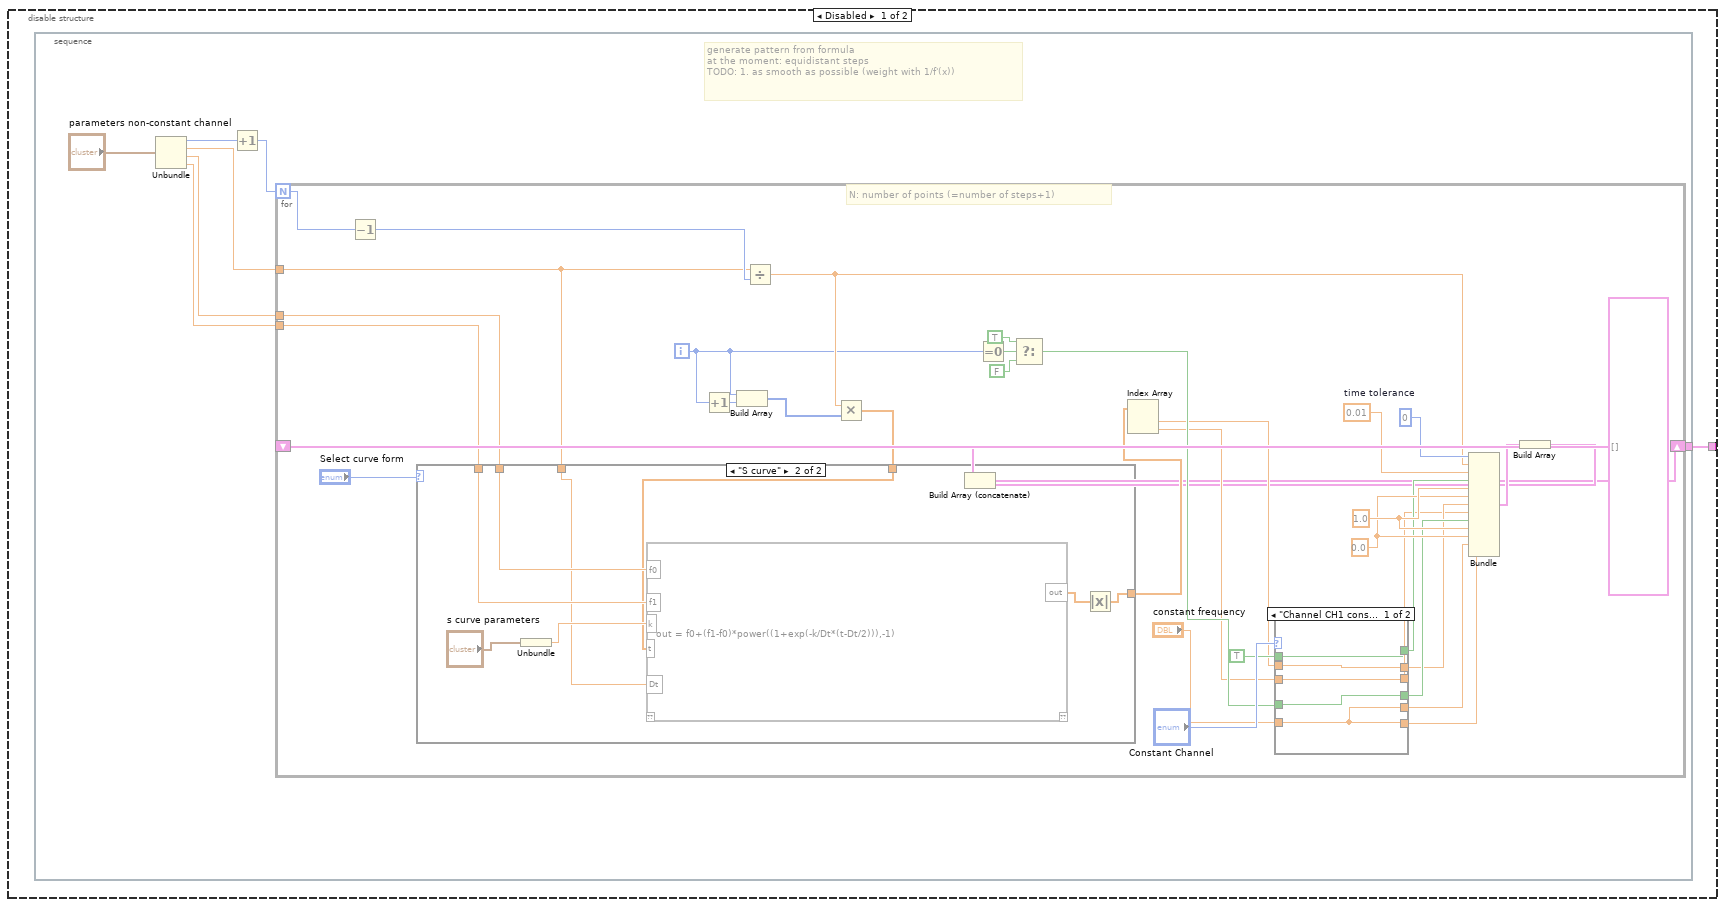
[diagram p2: hidden frame]
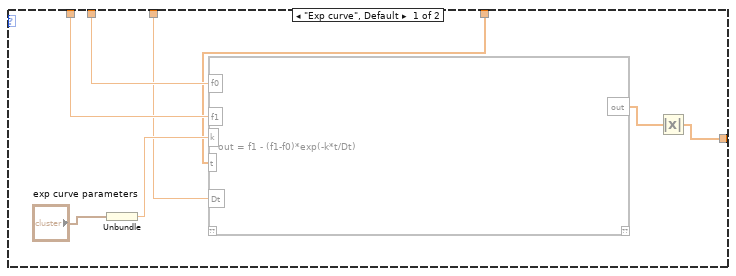
[diagram p4: hidden frame]
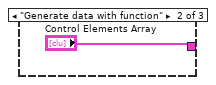
[diagram p5: hidden frame]
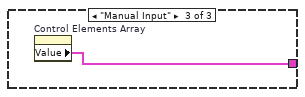
[diagram p6: hidden frame]
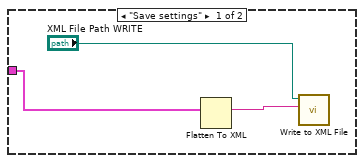
[diagram p7: hidden frame]
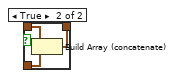
[diagram p8: hidden frame]
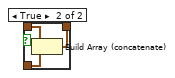
[diagram p9: hidden frame]
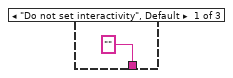
[diagram p10: hidden frame]
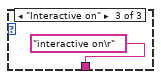
[diagram p11: hidden frame]
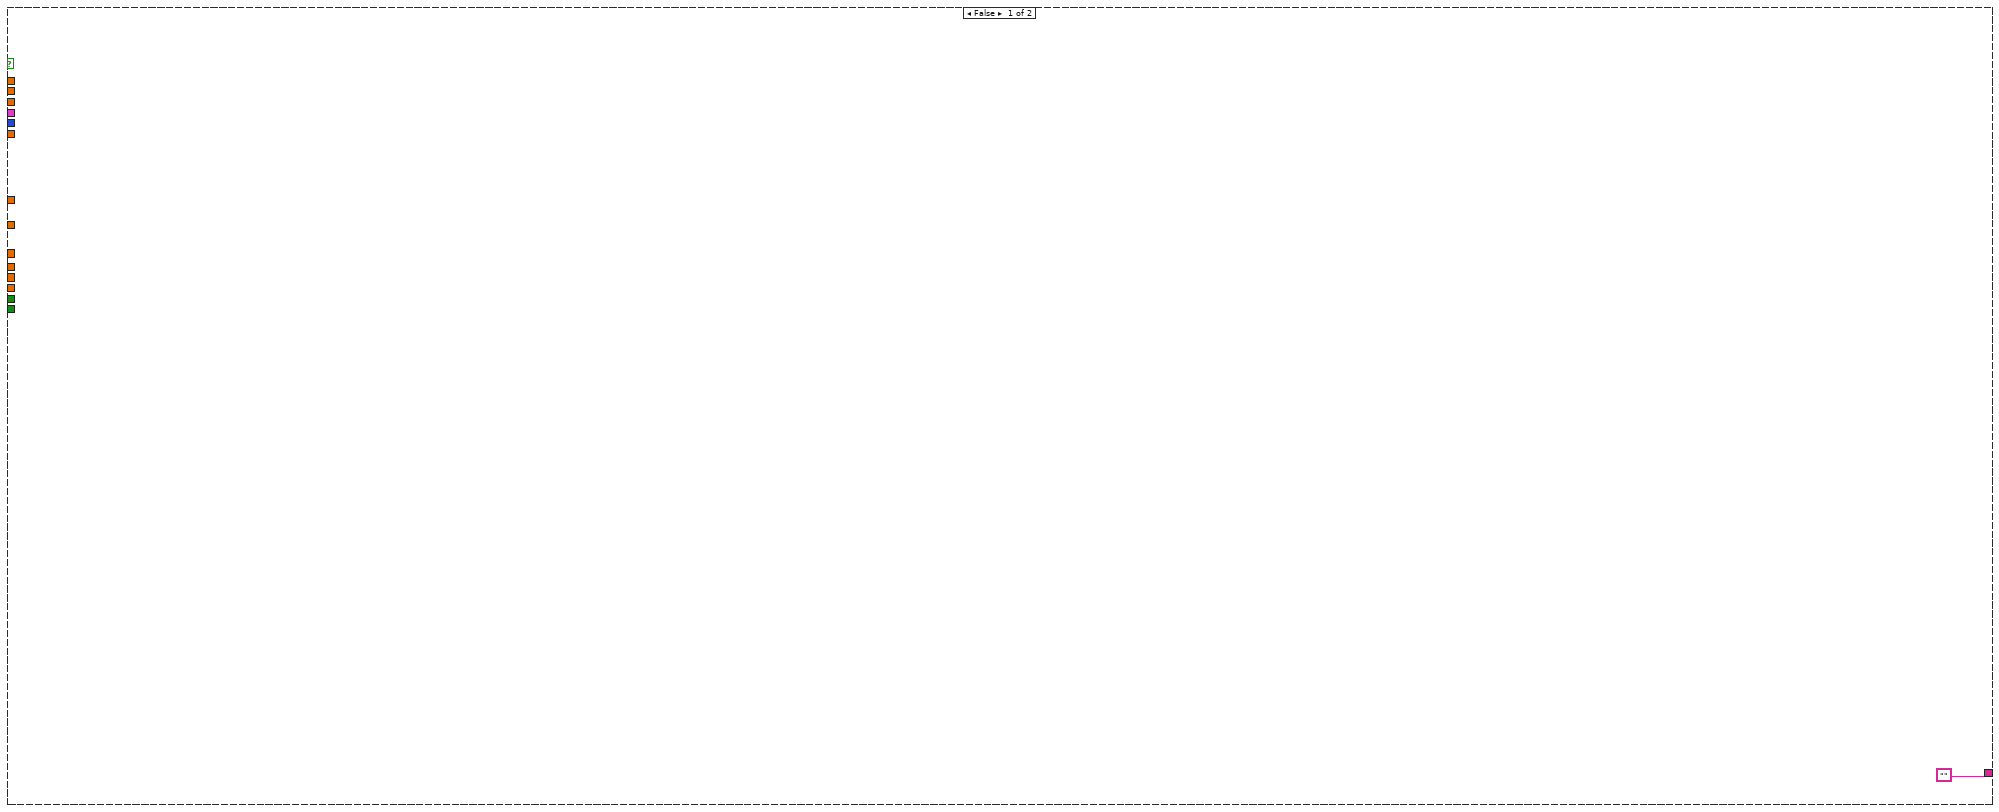
[diagram p12: hidden frame]
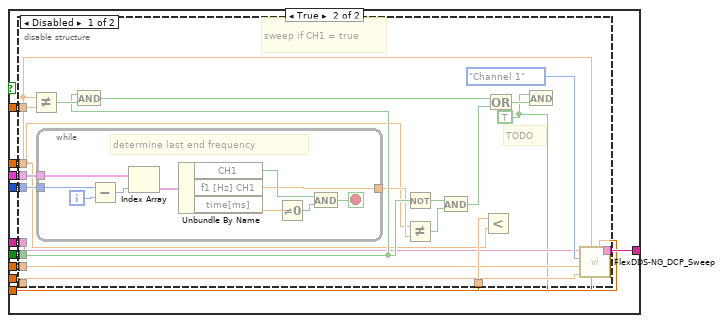
[diagram p13: hidden frame]
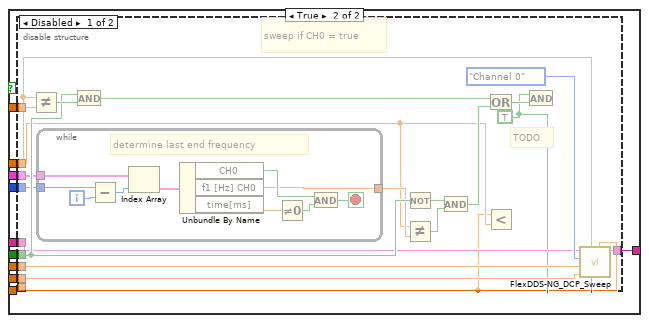
[diagram p15: hidden frame]
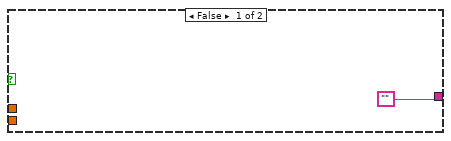
[diagram p18: hidden frame]
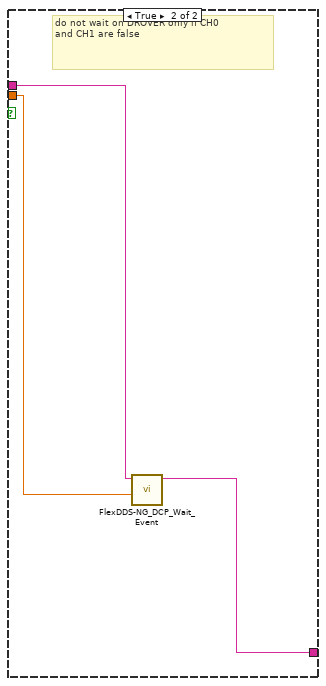
[diagram p19: hidden frame]
diagram:
  # "Relevant subvis for 'high level use':\nDCP Reset\nDCP Write STP\nDCP Write CFR1\nDCP Write CFR2\nDCP Write DRL\nDCP Write DRR\nDCP CMD (Bool)\nDCP Wait BNC\nDCP Wait Event\nDCP Start Stop\nTime To M/P\nDCP Sweep"
  n1 = disable-structure shown="Enabled" {
    disable-tunnel: [w23 _] -> w6
    frame Disabled {
      n2 = stacked-sequence {
        tunnel: [w30] -> w23
        frame #0 {
          # "generate pattern from formula\nat the moment: equidistant steps\nTODO: 1. as smooth as possible (weight with 1/f'(x))"
          n3 = Unbundle("parameters non-constant channel") -> ("Number of steps"=w29:i32, "time [ms]"=w27:dbl, "start frequency [Hz]"=w26:dbl, "end frequency [Hz]"=w25:dbl)
          n4 = Increment(x=w29) -> (x+1=w31:i32)
          n5 = for {
            N: w31 -> [w60]
            tunnel: w27 -> [w48]
            tunnel: w26 -> [w57]
            tunnel: w25 -> [w58]
            shift-right: [w32] -> w30
            shift-left: T10 [] -> [w33]
            i -> [w51]
            w63 = 1.0
            w62 = 0.0
            w64 = 0.01  # time tolerance
            # "N: number of points (=number of steps+1)"
            n6 = Decrement(x=w60) -> (x-1=w59:i32)
            n7 = Increment(x=w51) -> (x+1=w50:i32)
            n8 = Build Array(w51, w50) -> (w49:i32[])
            n9 = Divide(x=w48, y=w59) -> (x/y=w55:dbl)
            n10 = Multiply(x=w55, y=w49) -> (x*y=w56:dbl[])
            n11 = case shown="\"S curve\"" "Select curve form" {
              tunnel: w58 -> [w83 w90]
              tunnel: w57 -> [w84 w91]
              tunnel: w56 -> [w78 w88]
              tunnel: w48 -> [w79 w87]
              tunnel: [w77 w85] -> w47
              frame "Exp curve", Default {
                n12 = Unbundle("exp curve parameters") -> ("k"=w80:dbl)
                n13 = mathscript code="out = f1 - (f1-f0)*exp(-k*t/Dt)"("f0"=w84, "f1"=w83, "k"=w80, "t"=w78, "Dt"=w79) -> ("out"=w82:dbl[])  [unwired: 1 in, 1 out]
                n14 = Absolute Value(x=w82) -> (abs(x)=w77:dbl[])
              }
              frame "S curve" {
                n15 = Unbundle("s curve parameters") -> ("k"=w89:dbl)
                n16 = mathscript code="out = f0+(f1-f0)*power((1+exp(-k/Dt*(t-Dt/2))),-1)"("f0"=w91, "f1"=w90, "k"=w89, "t"=w88, "Dt"=w87) -> ("out"=w86:cdb[])  [unwired: 1 in, 1 out]
                n17 = Absolute Value(x=w86) -> (abs(x)=w85:dbl[])
              }
            }
            n18 = Equal To 0?(x=w51) -> (x = 0?=w54:bool)
            n19 = Select(t=TRUE, s=w54, f=FALSE) -> (s? t:f=w42:bool)
            n20 = Index Array(array=w47) -> (element #1=w38:dbl, element #2=w37:dbl)  [unwired: 2 in]
            n21 = case shown="\"Channel CH1 constant\", Default" "Constant Channel" {
              tunnel: "constant frequency" -> [w71 w72]
              tunnel: [w71 w74] -> w44
              tunnel: [w71 w75] -> w43
              tunnel: w42 -> [w70 w73]
              tunnel: [w70 w76] -> w41
              tunnel: TRUE -> [w69 w76]
              tunnel: [w69 w73] -> w39
              tunnel: w38 -> [w68 w75]
              tunnel: w37 -> [w67 w74]
              tunnel: [w68 w72] -> w36
              tunnel: [w67 w72] -> w35
              frame "Channel CH1 constant", Default {
              }
              frame "Channel CH0 constant" {
              }
            }
            n22 = Bundle(0, w55, "time tolerance"=w64, w39, w63, w62, "constant frequency"=w36, "constant frequency"=w35, w41, w63, w62, "constant frequency"=w43, "constant frequency"=w44) -> (w66:T11)  [unwired: 1 in]
            n23 = Build Array(w66) -> (w34:T10)
            n24 = Build Array (concatenate)(w33, w34) -> (w32:T10)
          }
        }
      }
    }
    frame Enabled {
    }
  }
  n25 = flat-sequence {
    tunnel: w6 -> [w93]
    tunnel: [w94] -> w5
    tunnel: w5 -> [w103]
    tunnel: [w103] -> w4
    tunnel: w4 -> [w109]
    tunnel: [w109] -> w3
    frame #0 {
      # "Input: read settings from xml file\nor generate data with function\nor use manual input from array"
      n26 = case shown="\"Read from file\"" "Data source" {
        tunnel: w93 -> [w97 _ _]
        tunnel: [w96 "Control Elements Array" w101] -> w94
        frame "Read from file" {
          n27 = call-poly <vilib>:"Read From XML File.vi"("XML File Path"="XML File Path READ") -> ("XML Elements"=w98:string)  [unwired: 8 in, 2 out]
          n28 = Unflatten From XML(xml string=w98, type=w97) -> (value=w96:T10)  [unwired: 1 in, 1 out]
          n29 = property on="Control Elements Array" class="Arr (strict)"("Value"=w96) -> ()  [unwired: 2 in, 2 out]
        }
        frame "Generate data with function" {
        }
        frame "Manual Input" {
          n30 = property on="Control Elements Array" class="Arr (strict)"() -> ("Value"=w101:T9)  [unwired: 2 in, 2 out]
        }
      }
    }
    frame #1 {
      # "save array/settings or don't save anything"
      n31 = case shown="\"Don't save settings\", Default" "Store data" {
        tunnel: w103 -> [w104 _]
        frame "Save settings" {
          n32 = Flatten To XML(anything=w104) -> (xml string=w106:string)
          n33 = call-poly <vilib>:"Write to XML File.vi"("XML Input"=w106, "XML File Path"="XML File Path WRITE") -> ()  [unwired: 7 in, 3 out]
        }
        frame "Don't save settings", Default {
        }
      }
    }
    frame #2 {
      w110 = 0.0  # total time[ms]
      # "plot frequency time plot AFTER reading"
      n34 = for {
        tunnel: w109 -> [w144] mode=indexing
        shift-right: [w143] -> _
        shift-left: w110 -> [w139]
        tunnel: w109 -> [w140]
        shift-right: [w118] -> w114
        shift-left: T13 [] ("Array") -> [w119]
        shift-right: [w116] -> w115
        shift-left: T12 [] ("Array") -> [w117]
        i -> [w141]
        # "iterate through linear ramps;\nif time==0: skip;\nif CHx==false: keep frequency;"
        n35 = flat-sequence {
          tunnel: w141 -> [w154]
          tunnel: w140 -> [w155]
          tunnel: [w156] -> w128
          tunnel: [w153] -> w127
          frame #0 {
            # "i: current index\nif CHx == false, look for largest index j<i with CHx=true (to determine which frequency to plot)"
            n36 = while {
              tunnel: w154 -> [w176]
              tunnel: w155 -> [w173]
              tunnel: [w171] -> w156
              i -> [w175]
              stop <- w169 stop-if-true
              n37 = Subtract(x=w176, y=w175) -> (x-y=w174:i32)
              n38 = Index Array(array=w173, index=w174) -> (element=w172:T14)
              n39 = Unbundle By Name(w172) -> ("f1 [Hz] CH0"=w171:dbl, "CH0"=w168:bool, "time[ms]"=w170:dbl)
              n40 = Not Equal To 0?(x=w170) -> (x != 0?=w167:bool)
              n41 = And(x=w168, y=w167) -> (x .and. y?=w169:bool)
            }
            n42 = while {
              tunnel: w154 -> [w166]
              tunnel: w155 -> [w163]
              tunnel: [w161] -> w153
              i -> [w165]
              stop <- w159 stop-if-true
              n43 = Subtract(x=w166, y=w165) -> (x-y=w164:i32)
              n44 = Index Array(array=w163, index=w164) -> (element=w162:T14)
              n45 = Unbundle By Name(w162) -> ("f1 [Hz] CH1"=w161:dbl, "CH1"=w158:bool, "time[ms]"=w160:dbl)
              n46 = Not Equal To 0?(x=w160) -> (x != 0?=w157:bool)
              n47 = And(x=w158, y=w157) -> (x .and. y?=w159:bool)
            }
          }
        }
        n48 = Unbundle By Name(w144) -> ("time[ms]"=w142:dbl, "f0 [Hz] CH0"=w132:dbl, "f1 [Hz] CH0"=w131:dbl, "f0 [Hz] CH1"=w130:dbl, "f1 [Hz] CH1"=w129:dbl, "CH0"=w134:bool, "CH1"=w133:bool)
        n49 = Add(x=w139, y=w142) -> (x+y=w143:dbl)
        n50 = Not Equal To 0?(x=w142) -> (x != 0?=w120:bool)
        n51 = Select(t=w132, s=w134, f=w128) -> (s? t:f=w136:dbl)
        n52 = Select(t=w131, s=w134, f=w128) -> (s? t:f=w135:dbl)
        n53 = Select(t=w130, s=w133, f=w127) -> (s? t:f=w138:dbl)
        n54 = Select(t=w129, s=w133, f=w127) -> (s? t:f=w137:dbl)
        n55 = Bundle("total time[ms]"=w139, "f1 [Hz] CH0"=w136) -> (w126:cluster{"total time[ms]":dbl, "f1 [Hz] CH0":dbl})  [unwired: 1 in]
        n56 = Bundle(w143, "f1 [Hz] CH0"=w135) -> (w125:cluster{dbl, "f1 [Hz] CH0":dbl})  [unwired: 1 in]
        n57 = Bundle("total time[ms]"=w139, "f1 [Hz] CH1"=w138) -> (w124:cluster{"total time[ms]":dbl, "f1 [Hz] CH1":dbl})  [unwired: 1 in]
        n58 = Bundle(w143, "f1 [Hz] CH1"=w137) -> (w123:cluster{dbl, "f1 [Hz] CH1":dbl})  [unwired: 1 in]
        n59 = Build Array(w126, w125) -> (w122:T13)
        n60 = case shown="False" w120 {
          tunnel: w119 -> [w149 w151]
          tunnel: w122 -> [_ w150]
          tunnel: [w149 w152] -> w118
          frame False {
          }
          frame True {
            n61 = Build Array (concatenate)(w151, w150) -> (w152:T13)
          }
        }
        n62 = Build Array(w124, w123) -> (w121:T12)
        n63 = case shown="False" w120 {
          tunnel: w117 -> [w145 w147]
          tunnel: w121 -> [_ w146]
          tunnel: [w145 w148] -> w116
          frame False {
          }
          frame True {
            n64 = Build Array (concatenate)(w147, w146) -> (w148:T12)
          }
        }
      }
      n65 = Bundle("Array"=w114) -> (w111:T15)  [unwired: 1 in]
      n66 = Bundle("Array"=w115) -> (w112:T16)  [unwired: 1 in]
      n67 = Build Array(w111, w112) -> (→"frequency-time plot":T17)
    }
  }
  n68 = flat-sequence {
    frame #0 {
      # "This is the central data structure, work with property nodes to simplify reading and writing settings"
    }
  }
  n69 = flat-sequence {
    tunnel: [w182] -> w13
    tunnel: [w180] -> w12
    tunnel: w3 -> [w180]
    tunnel: w13 -> [w191]
    tunnel: w12 -> [w186]
    tunnel: [w189] -> w10
    tunnel: [w186] -> w8
    tunnel: w10 -> [w194]
    tunnel: [w193] -> w9
    tunnel: w8 -> [w197]
    tunnel: [w197] -> w7
    tunnel: w9 -> [w198]
    tunnel: w7 -> [w202]
    tunnel: [w200] -> w11
    tunnel: [w449] -> w1
    tunnel: w11 -> [w448]
    frame #0 {
      # "Interactive off + Full Reset"
      n70 = case shown="\"Interactive off\"" "Interactive on/off" {
        tunnel: ["" ("input 1") "interactive off\r" ("input 1") "interactive on\r" ("input 1")] -> w177
        frame "Do not set interactivity", Default {
        }
        frame "Interactive off" {
        }
        frame "Interactive on" {
        }
      }
      n71 = Format Into String(w177) -> (resulting string=w179:string)  [unwired: 3 in, 1 out]
      n72 = call "FlexDDS-NG_DCP_Reset.vi"("full reset (yes)"=TRUE, "initial instruction string"=w179) -> ("appended instruction string"=w182:string)  [unwired: 9 in]
    }
    frame #1 {
      w190 = T18."Both channels" ("Channels")
      # "* inverse sinc filter\n* digital ramp enable\n* matched latency enable"
      # "Write CFR1 and CFR2"
      n73 = call "FlexDDS-NG_DCP_WriteCFR1_C.vi"("CFR1 bits"="CFR1 bits", "Channels"=w190, "initial instruction string"=w191) -> ("appended instruction string"=w192:string)  [unwired: 8 in]
      n74 = call "FlexDDS-NG_DCP_WriteCFR2_C.vi"("CFR2 bits"="CFR2 bits", "Channels"=w190, "initial instruction string"=w192) -> ("appended instruction string"=w189:string)  [unwired: 8 in]
    }
    frame #2 {
      # "add trigger"
      n75 = call "FlexDDS-NG_DCP_Wait_BNC.vi"("Trigger"="Trigger before sequence of sweeps", "Channels"=T18."Both channels" ("Channels 2"), "appended instruction string in"=w194) -> ("appended instruction string"=w193:string)  [unwired: 8 in]
    }
    frame #3 {
      # "iterate through array of clusters and create command string\nif 1st command is decreasing ramp add very short increasing ramp before\nignore all columns with time=0ms\nTODO: write some detailed documentation what is going on below"
      n76 = Array Size(array=w202) -> (size(s)=w203:i32)
      n77 = for {
        N: w203 -> [_]
        tunnel: w202 -> [w233] mode=indexing
        tunnel: w202 -> [w219]
        tunnel: [w232] -> w201 mode=indexing
        i -> [w231]
        # "iterate through array of time steps"
        n78 = Unbundle(w233) -> ("time[ms]"=w225:dbl, "time tolerance[us]"=w224:dbl, "CH0"=w230:bool, "rel. amplitude CH0"=w223:dbl, "phase [°] CH0"=w222:dbl, "f0 [Hz] CH0"=w229:dbl, "f1 [Hz] CH0"=w228:dbl, "CH1"=w204:bool, "rel. amplitude CH1"=w221:dbl, "phase [°] CH1"=w220:dbl, "f0 [Hz] CH1"=w227:dbl, "f1 [Hz] CH1"=w226:dbl)  [unwired: 1 out]
        n79 = flat-sequence {
          tunnel: w219 -> [w281]
          tunnel: w220 -> [w245]
          tunnel: w221 -> [w246]
          tunnel: w222 -> [w249]
          tunnel: w223 -> [w250]
          tunnel: w224 -> [w282]
          tunnel: w225 -> [w236]
          tunnel: w226 -> [w243]
          tunnel: w227 -> [w244]
          tunnel: w228 -> [w247]
          tunnel: w229 -> [w248]
          tunnel: w230 -> [w254]
          tunnel: w231 -> [w241]
          tunnel: [w241] -> w218
          tunnel: [w254] -> w217
          tunnel: [w251] -> w216
          tunnel: [w248] -> w215
          tunnel: [w247] -> w214
          tunnel: [w244] -> w213
          tunnel: [w243] -> w212
          tunnel: [w236] -> w211
          tunnel: [w282] -> w210
          tunnel: [w250] -> w209
          tunnel: [w249] -> w208
          tunnel: [w246] -> w207
          tunnel: [w245] -> w206
          tunnel: [w281] -> w205
          tunnel: w204 -> [w251]
          tunnel: [w297] -> w232
          tunnel: w218 -> [w296]
          tunnel: w217 -> [w295]
          tunnel: w216 -> [w294]
          tunnel: w215 -> [w284]
          tunnel: w214 -> [w283]
          tunnel: w213 -> [w293]
          tunnel: w212 -> [w292]
          tunnel: w211 -> [w291]
          tunnel: w210 -> [w285]
          tunnel: w209 -> [w290]
          tunnel: w208 -> [w289]
          tunnel: w207 -> [w288]
          tunnel: w206 -> [w287]
          tunnel: w205 -> [w286]
          frame #0 {
            # "0<=ampl<=1\n0<=freq<=400MHz\n0<=phase=360\nChx[0] not FALSE\ntime[0] not 0"
            # "check if input is valid\nabort otherwise"
            n80 = Equal To 0?(x=w241) -> (x = 0?=w238:bool)
            n81 = Equal To 0?(x=w236) -> (x = 0?=w237:bool)
            n82 = In Range and Coerce(upper limit=360.0, x=w249, lower limit=0.0) -> (In Range?=w261:bool)  [unwired: 1 out]
            n83 = In Range and Coerce(upper limit=360.0, x=w245, lower limit=0.0) -> (In Range?=w260:bool)  [unwired: 1 out]
            n84 = And(x=w238, y=w237) -> (x .and. y?=w235:bool)
            n85 = Not(x=w235) -> (.not. x?=w234:bool)
            n86 = Select(t=w254, s=w238, f=TRUE) -> (s? t:f=w256:bool)
            n87 = Select(t=w251, s=w238, f=TRUE) -> (s? t:f=w252:bool)
            n88 = In Range and Coerce(upper limit=400000000.0, x=w248, lower limit=0.0) -> (In Range?=w265:bool)  [unwired: 1 out]
            n89 = In Range and Coerce(upper limit=400000000.0, x=w247, lower limit=0.0) -> (In Range?=w264:bool)  [unwired: 1 out]
            n90 = In Range and Coerce(upper limit=400000000.0, x=w244, lower limit=0.0) -> (In Range?=w263:bool)  [unwired: 1 out]
            n91 = In Range and Coerce(upper limit=400000000.0, x=w243, lower limit=0.0) -> (In Range?=w262:bool)  [unwired: 1 out]
            n92 = In Range and Coerce(upper limit=1.0, x=w250, lower limit=0.0) -> (In Range?=w259:bool)  [unwired: 1 out]
            n93 = In Range and Coerce(upper limit=1.0, x=w246, lower limit=0.0) -> (In Range?=w258:bool)  [unwired: 1 out]
            n94 = Compound Arithmetic op=AND(w265, w264, w263, w262, w261, w260, w259, w258, w256, w252, w234) -> (w242:bool)
            n95 = Not(x=w242) -> (.not. x?=w240:bool)
            n96 = call "Display Message to User"("Enable"=w240) -> ("OK"=w239:bool)  [unwired: 9 in, 1 out]
            n97 = Stop(stop? (T)=w239) -> ()
          }
          frame #1 {
            n98 = Not Equal?(x=0.0, y=w291) -> (x != y?=w298:bool)
            n99 = case shown="True" w298 {
              tunnel: ["" w342] -> w297
              tunnel: w296 -> [_ w308]
              tunnel: w295 -> [_ w319]
              tunnel: w294 -> [_ w311]
              tunnel: w291 -> [_ w303]
              tunnel: w293 -> [_ w310]
              tunnel: w292 -> [_ w301]
              tunnel: w290 -> [_ w323]
              tunnel: w289 -> [_ w331]
              tunnel: w288 -> [_ w330]
              tunnel: w287 -> [_ w329]
              tunnel: w286 -> [_ w309]
              tunnel: w285 -> [_ w302]
              tunnel: w284 -> [_ w316]
              tunnel: w283 -> [_ w315]
              frame False {
              }
              frame True {
                # "1st iteration and amplitude or phase changed"
                # "skip if time is zero"
                n100 = Decrement(x=w308) -> (x-1=w341:i32)
                n101 = Not(x=w319) -> (.not. x?=w344:bool)
                n102 = Not(x=w311) -> (.not. x?=w343:bool)
                n103 = And(x=w344, y=w343) -> (x .and. y?=w345:bool)
                n104 = Index Array(array=w309, index=w341) -> (element=w314:T14)
                n105 = Unbundle By Name(w314) -> ("rel. amplitude CH0"=w337:dbl, "phase [°] CH0"=w336:dbl, "rel. amplitude CH1"=w333:dbl, "phase [°] CH1"=w332:dbl)
                n106 = Unbundle By Name(w314) -> ("CH0"=w312:bool, "CH1"=w305:bool, "f1 [Hz] CH0"=w313:dbl, "f1 [Hz] CH1"=w304:dbl)
                n107 = Equal?(x=w323, y=w337) -> (x = y?=w338:bool)
                n108 = Equal?(x=w331, y=w336) -> (x = y?=w339:bool)
                n109 = Equal?(x=w333, y=w330) -> (x = y?=w335:bool)
                n110 = And(x=w338, y=w339) -> (x .and. y?=w327:bool)
                n111 = Not(x=w327) -> (.not. x?=w326:bool)
                n112 = Equal To 0?(x=w308) -> (x = 0?=w340:bool)
                n113 = Or(x=w340, y=w326) -> (x .or. y?=w320:bool)
                n114 = And(x=w319, y=w320) -> (x .and. y?=w317:bool)
                n115 = case shown="True" w317 {
                  tunnel: w323 -> [_ w436]
                  tunnel: w331 -> [_ w435]
                  tunnel: ["" w434] -> w328
                  frame False {
                  }
                  frame True {
                    # "CH0: write stp if (i==0 or ampl/phase changed) and CH0 = true"
                    n116 = call "FlexDDS-NG_DCP_WriteSTP.vi"("phase degrees (0..360)"=w435, "amplitude (0..1)"=w436, "Channels"=T18."Channel 0", "initial instruction string"="") -> ("appended instruction string"=w434:string)  [unwired: 7 in]
                  }
                }
                n117 = Equal?(x=w332, y=w329) -> (x = y?=w334:bool)
                n118 = And(x=w335, y=w334) -> (x .and. y?=w325:bool)
                n119 = Not(x=w325) -> (.not. x?=w324:bool)
                n120 = Or(x=w340, y=w324) -> (x .or. y?=w321:bool)
                n121 = And(x=w311, y=w321) -> (x .and. y?=w318:bool)
                n122 = case shown="True" w318 {
                  tunnel: [w426 w431] -> w322
                  tunnel: w330 -> [_ w429]
                  tunnel: w329 -> [_ w428]
                  tunnel: w328 -> [w426 w427]
                  frame False {
                  }
                  frame True {
                    # "CH1: write stp if (i==0 or ampl/phase changed) and CH1 = true"
                    n123 = call "FlexDDS-NG_DCP_WriteSTP.vi"("phase degrees (0..360)"=w428, "amplitude (0..1)"=w429, "Channels"=T18."Channel 1", "initial instruction string"=w427) -> ("appended instruction string"=w431:string)  [unwired: 7 in]
                  }
                }
                n124 = case shown="False" w319 {
                  tunnel: w322 -> [w386 w392]
                  tunnel: [w386 w391] -> w307
                  tunnel: w303 -> [_ w389]
                  tunnel: w302 -> [_ w388]
                  tunnel: w316 -> [_ w390]
                  tunnel: w315 -> [_ w387]
                  tunnel: w313 -> [_ w396]
                  tunnel: w312 -> [_ w395]
                  tunnel: w309 -> [_ w394]
                  tunnel: w308 -> [_ w393]
                  frame False {
                  }
                  frame True {
                    n125 = disable-structure shown="Disabled" {
                      disable-tunnel: w396 -> [w414 _]
                      disable-tunnel: w395 -> [w409 _]
                      disable-tunnel: w394 -> [w407 _]
                      disable-tunnel: w393 -> [w406 _]
                      disable-tunnel: w392 -> [w403 _]
                      disable-tunnel: [w402 _] -> w391
                      disable-tunnel: w390 -> [w401 _]
                      disable-tunnel: w389 -> [w400 _]
                      disable-tunnel: w388 -> [w399 _]
                      disable-tunnel: w387 -> [w397 _]
                      frame Disabled {
                        w398 = TRUE ("x")
                        # "TODO"
                        # "sweep if CH0 = true"
                        n126 = Not Equal?(x=w401, y=w414) -> (x != y?=w412:bool)
                        n127 = while {
                          tunnel: w407 -> [w425]
                          tunnel: w406 -> [w423]
                          tunnel: [w416] -> w405
                          i -> [w424]
                          stop <- w417 stop-if-true
                          # "determine last end frequency"
                          n128 = Subtract(x=w423, y=w424) -> (x-y=w422:i32)
                          n129 = Index Array(array=w425, index=w422) -> (element=w421:T14)
                          n130 = Unbundle By Name(w421) -> ("CH0"=w418:bool, "f1 [Hz] CH0"=w416:dbl, "time[ms]"=w420:dbl)
                          n131 = Not Equal To 0?(x=w420) -> (x != 0?=w419:bool)
                          n132 = And(x=w418, y=w419) -> (x .and. y?=w417:bool)
                        }
                        n133 = And(x=w409, y=w412) -> (x .and. y?=w413:bool)
                        n134 = Not(x=w409) -> (.not. x?=w410:bool)
                        n135 = Not Equal?(x=w401, y=w405) -> (x != y?=w408:bool)
                        n136 = And(x=w410, y=w408) -> (x .and. y?=w411:bool)
                        n137 = Or(x=w413, y=w411) -> (x .or. y?=w415:bool)
                        n138 = Less?(x=w397, y=w401) -> ()  [unwired: 1 out]
                        n139 = And(x=w398, y=w415) -> ()  [unwired: 1 out]
                        n140 = call "FlexDDS-NG_DCP_Sweep.vi"("f1"=w397, "jump before ramp"=w398, "f0"=w401, "sweep time tolerance (us)"=w399, "sweep time (ms)"=w400, "Channels in"=T18."Channel 0", "initial instruction string"=w403) -> ("appended instruction string out"=w402:string)  [unwired: 4 in]
                      }
                      frame Enabled {
                      }
                    }
                  }
                }
                n141 = case shown="False" w311 {
                  tunnel: w307 -> [w346 w351]
                  tunnel: [w346 w350] -> w306
                  tunnel: w303 -> [_ w348]
                  tunnel: w302 -> [_ w347]
                  tunnel: w310 -> [_ w349]
                  tunnel: w301 -> [_ w352]
                  tunnel: w304 -> [_ w356]
                  tunnel: w305 -> [_ w355]
                  tunnel: w309 -> [_ w354]
                  tunnel: w308 -> [_ w353]
                  frame False {
                  }
                  frame True {
                    n142 = disable-structure shown="Disabled" {
                      disable-tunnel: w356 -> [w374 _]
                      disable-tunnel: w355 -> [w369 _]
                      disable-tunnel: w354 -> [w367 _]
                      disable-tunnel: w353 -> [w366 _]
                      disable-tunnel: w352 -> [w363 _]
                      disable-tunnel: w351 -> [w362 _]
                      disable-tunnel: [w361 _] -> w350
                      disable-tunnel: w349 -> [w360 _]
                      disable-tunnel: w348 -> [w359 _]
                      disable-tunnel: w347 -> [w358 _]
                      frame Disabled {
                        w357 = TRUE ("x")
                        # "TODO"
                        # "sweep if CH1 = true"
                        n143 = Not Equal?(x=w360, y=w374) -> (x != y?=w372:bool)
                        n144 = while {
                          tunnel: w367 -> [w385]
                          tunnel: w366 -> [w383]
                          tunnel: [w376] -> w365
                          i -> [w384]
                          stop <- w377 stop-if-true
                          # "determine last end frequency"
                          n145 = Subtract(x=w383, y=w384) -> (x-y=w382:i32)
                          n146 = Index Array(array=w385, index=w382) -> (element=w381:T14)
                          n147 = Unbundle By Name(w381) -> ("CH1"=w378:bool, "f1 [Hz] CH1"=w376:dbl, "time[ms]"=w380:dbl)
                          n148 = Not Equal To 0?(x=w380) -> (x != 0?=w379:bool)
                          n149 = And(x=w378, y=w379) -> (x .and. y?=w377:bool)
                        }
                        n150 = And(x=w369, y=w372) -> (x .and. y?=w373:bool)
                        n151 = Not(x=w369) -> (.not. x?=w370:bool)
                        n152 = Not Equal?(x=w360, y=w365) -> (x != y?=w368:bool)
                        n153 = And(x=w370, y=w368) -> (x .and. y?=w371:bool)
                        n154 = Less?(x=w363, y=w360) -> ()  [unwired: 1 out]
                        n155 = Or(x=w373, y=w371) -> (x .or. y?=w375:bool)
                        n156 = And(x=w357, y=w375) -> ()  [unwired: 1 out]
                        n157 = call "FlexDDS-NG_DCP_Sweep.vi"("f1"=w363, "jump before ramp"=w357, "f0"=w360, "sweep time tolerance (us)"=w358, "sweep time (ms)"=w359, "Channels in"=T18."Channel 1", "initial instruction string"=w362) -> ("appended instruction string out"=w361:string)  [unwired: 4 in]
                      }
                      frame Enabled {
                      }
                    }
                  }
                }
                n158 = case shown="False" w345 {
                  tunnel: [w439 w447] -> w342
                  tunnel: w303 -> [_ w446]
                  tunnel: w306 -> [w438 w445]
                  frame False {
                    # "wait on DROVER if one of the channels\nwait 8ns (1h) before waiting on DROVER"
                    n159 = call "FlexDDS-NG_DCP_Wait_Event.vi"("waiting time [ms]"=8e-06, "Channels in"=T18."Both channels", "appended instruction string in"=w438) -> ("appended instruction string"=w440:string)  [unwired: 8 in]
                    n160 = call "FlexDDS-NG_DCP_Wait_Event.vi"("Event 1"=T19."DROVER", "Channels in"=T18."Both channels", "appended instruction string in"=w440) -> ("appended instruction string"=w439:string)  [unwired: 8 in]
                  }
                  frame True {
                    # "do not wait on DROVER only if CH0\nand CH1 are false"
                    n161 = call "FlexDDS-NG_DCP_Wait_Event.vi"("waiting time [ms]"=w446, "appended instruction string in"=w445) -> ("appended instruction string"=w447:string)  [unwired: 9 in]
                  }
                }
              }
            }
          }
        }
      }
      n162 = Concatenate Strings(w201) -> (w199:string)
      n163 = Format Into String(initial string=w198, w199) -> (resulting string=w200:string)  [unwired: 2 in, 1 out]
    }
    frame #4 {
      # "start"
      n164 = call "FlexDDS-NG_DCP_StartStop.vi"("initial instruction string"=w448) -> ("appended instruction string"=w449:string)  [unwired: 10 in]
    }
  }
  n165 = call "FlexDDS-NG_USB_VISA_Open.vi"("FlexDDS-NG USB VISA resource name (COM)"="FlexDDS-NG USB VISA resource name (COM)") -> ("error out"=w15:errorcluster, "FlexDDS-NG USB VISA resource name out"=w17:refnum<visa-resource-name>)  [unwired: 9 in]
  n166 = VISA Write(VISA resource name=w17, write buffer=w1, error in (no error)=w15) -> (VISA resource name out=w18:refnum<visa-resource-name>, return count=→"return count":u32, error out=w14:errorcluster)
  n167 = VISA Read(VISA resource name=w18, byte count=u32 500, error in (no error)=w14) -> (VISA resource name out=w21:refnum<visa-resource-name>, read buffer=→"read buffer":string, error out=→"error out":errorcluster)  [unwired: 1 out]
  n168 = VISA Close(VISA resource name=w21) -> ()  [unwired: 1 in, 1 out]
  "appended instruction string 4" <- w1
